vi "Off Mode Standby Mode Power Measure SM.vi"(0 "Equipment":T3, 1 "CDAQ Tasks":refnum<k21>[](array[refnum]), 11 "Error In":errorcluster) -> (4 "Off Mode Watts":dbl, 6 "2015 Output":bool, 8 "Standby Watts":dbl, 10 "Low Power Switch":bool=TRUE, 15 "Error Out":errorcluster)   [LabVIEW 2013]
uses:
  Type Definitions/Equipment DPT.ctl
  Type Definitions/WT500 Sequences.ctl
  <vilib>/Analysis/NI_AALBase.lvlib
panel:
  in  "Main Tab":enum32{"Collecting", "Analyzed"}(tab)
  in  "stop":bool
  out "Power Chart":dbl(graph)
  out "Power (Watts)":dbl
  in  "Skip Standby":bool
  in  "2015 DOE":bool
  out "Off Mode Watts":T1(graph)
  out "5% of Max.":dbl
  out "Max Value.":dbl
  out "Standard Deviation.":dbl
  out "Standby Mode Watts":T1(graph)
  out "Standard Deviation":dbl
  out "Max Value":dbl
  out "5% of Max":dbl
  in  "Complete Test":bool
  in  "Restart":bool
  out "Stable?":bool
  out "Time Sum 4":dbl
  out "Time Sum 3":dbl
  out "Time Sum 2":dbl
  out "Time Sum 1":dbl
  in  "Tab Control":enum32{"Input Parameters", "Debug", "Raw Data"}(tab)
  in  "Processed Data":bool
  in  "Tab Control 2":T2(tab)
  in  "10 Min Power":dbl=600.0
  in  "35 Min":dbl=2100.0
  in  "5 Min Timer":dbl=300.0
  in  "2015?":bool
  out "Current State":string
  in  "High State Timer":dbl=10.0
  out "High Power":dbl
  in  "Low State Timer (5 min)":dbl=300.0
  out "Power Threshold":dbl
  in  "Testing":bool
  in  "Test Power":dbl
  in  "Debug?":bool=TRUE
  out "Debug State":string[](array[string])
  out "DOE Data":dbl[][](array[numeric])
  out "35 Min Data":dbl[][](array[numeric])
  out "Power Threshold Array":dbl[][](array[numeric])
  out "Timer":dbl format="%<%H:%M:%S>t"
  out "String":string
  # "Measure off mode and standby mode for DOE 2015. Reference ETP 112D026 - 2015 DOE Dryer Energy"
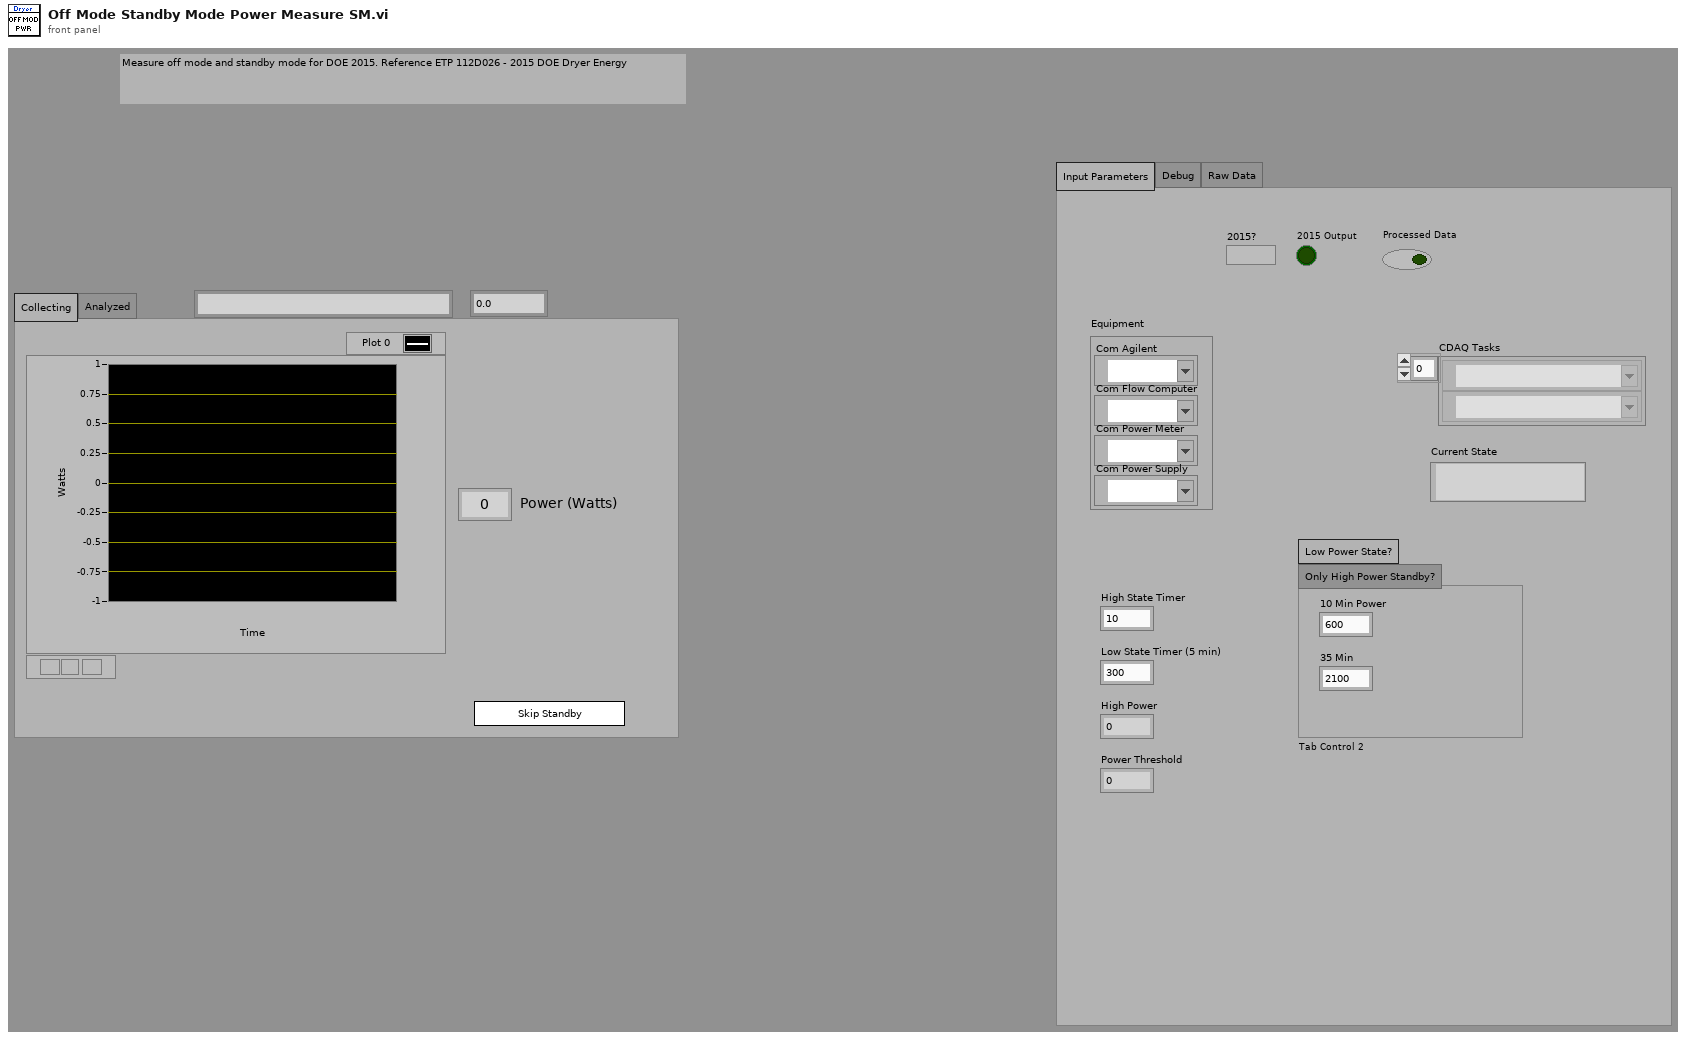
[diagram p1: front panel]
types:
  T1 = cluster{"X Values":dbl[], "Histogram: h(x)":i32[]}
  T2 = enum32{"Low Power State?", "Only High Power Standby?"}
  T3 = typedef "Equipment DPT.ctl" = cluster{"Com Agilent":refnum<visa-resource-name>, "Com Flow Computer":refnum<visa-resource-name>, "Com Power Meter":refnum<visa-resource-name>, "Com Power Supply":refnum<visa-resource-name>}
  T4 = enum32{"invalid app kind", "Development System", "Run Time System", "Student Edition", "Embedded LabVIEW", "Evaluation", "Custom"}
  T5 = enum16{"Exe", "Init CDAQ", "Gather DATA", "Close"}
  T6 = enum32{"Invalid", "Standard", "Closed", "Hidden", "Minimized", "Maximized"}
  T7 = typedef "WT500 Sequences.ctl" = enum16{"Initialize", "GetReadings", "GetErrors", "Close", "NoOp", "MiscCmd"}
  T8 = cluster{"Core":cluster{"Current VI Reference":refnum<vi>, "Close Panel on Exit?":bool}, "Agilent Channel List":string, "Equipment":T3, "T0":dbl, "Tstart":dbl, "Temps":dbl[], "2015?":bool, "CDAQ Tasks":refnum<k21>[], "Labels":string[], "35 Min Data Array":dbl[], "10 Min Data Array":dbl[], "Low Power State?":bool, "Output Data":cluster{"Standard Deviation":dbl, "Off Mode Watts":dbl, "Max Value":dbl, "5% of Max":dbl, "Standby Watts":dbl, "Standard Deviation.":dbl, "Max Value.":dbl, "5% of Max.":dbl}, "Power Threshold":dbl[], "Processed Data":bool, "Main Tab":enum32{"Collecting", "Analyzed"}}
  T9 = cluster{"Standard Deviation":dbl, "Off Mode Watts":dbl, "Max Value":dbl, "5% of Max":dbl, "Standby Watts":dbl, "Standard Deviation.":dbl, "Max Value.":dbl, "5% of Max.":dbl}
  T10 = cluster{"Current VI Reference":refnum<vi>, "Close Panel on Exit?":bool}
  T11 = typedef "Dryer PowerData.ctl" = cluster{"Current L1":dbl, "Current L2":dbl, "Power":dbl, "WattHours":dbl}
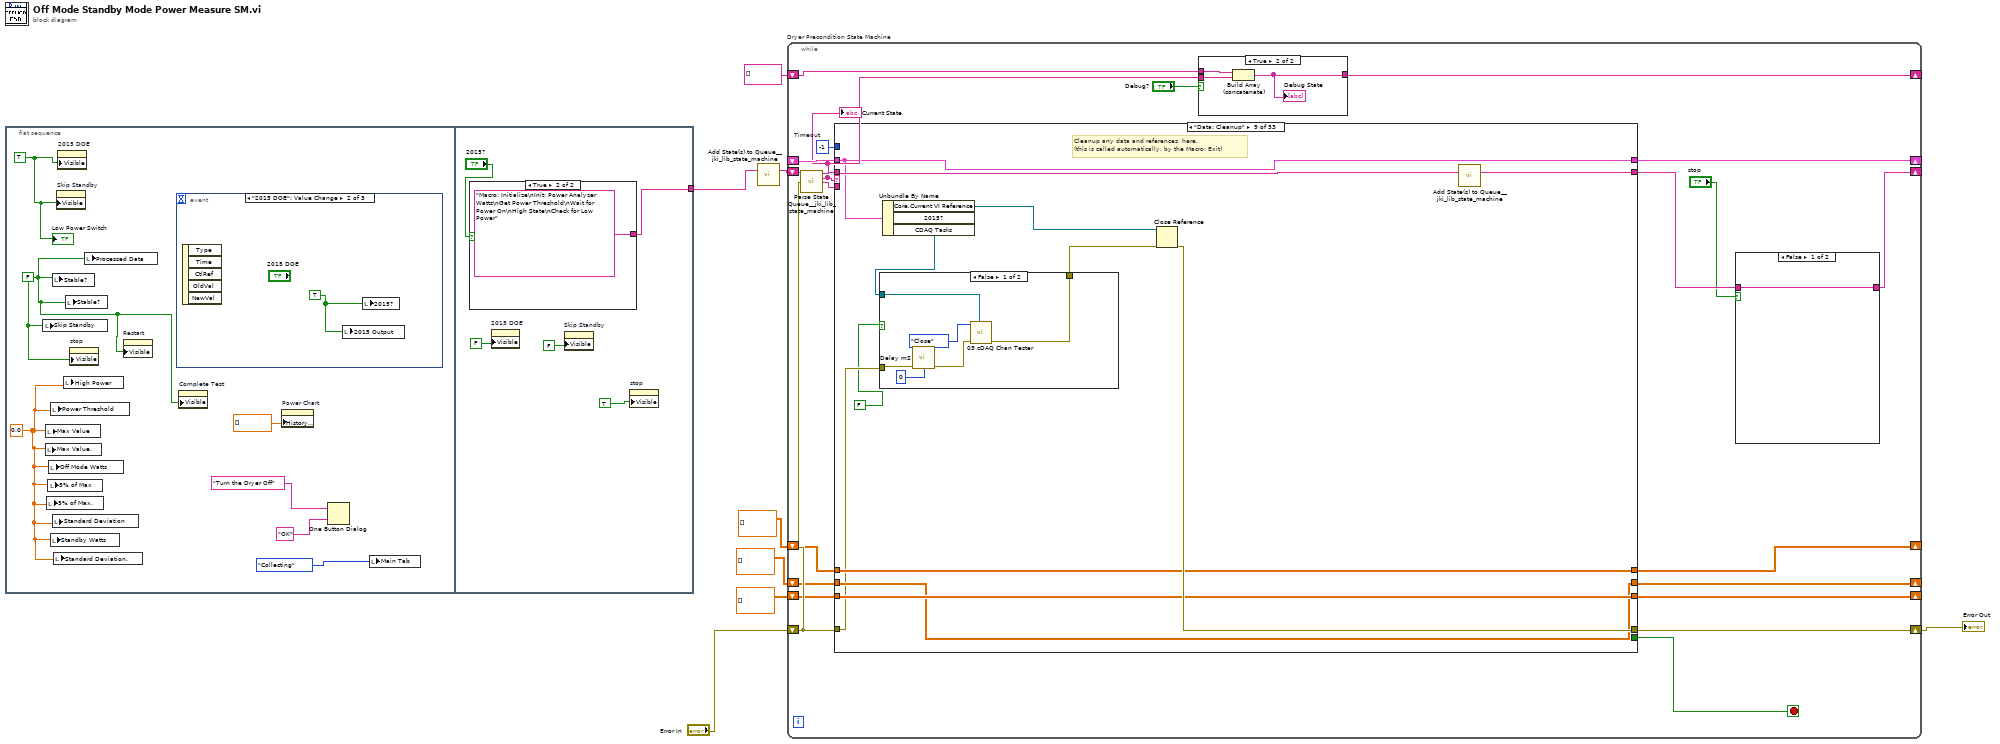
[diagram p0: block diagram]
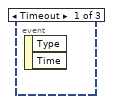
[diagram p2: hidden frame]
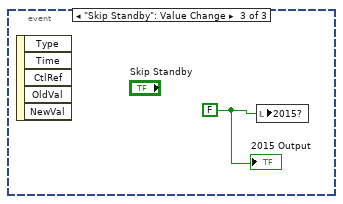
[diagram p3: hidden frame]
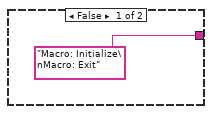
[diagram p4: hidden frame]
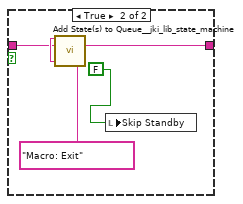
[diagram p5: hidden frame]
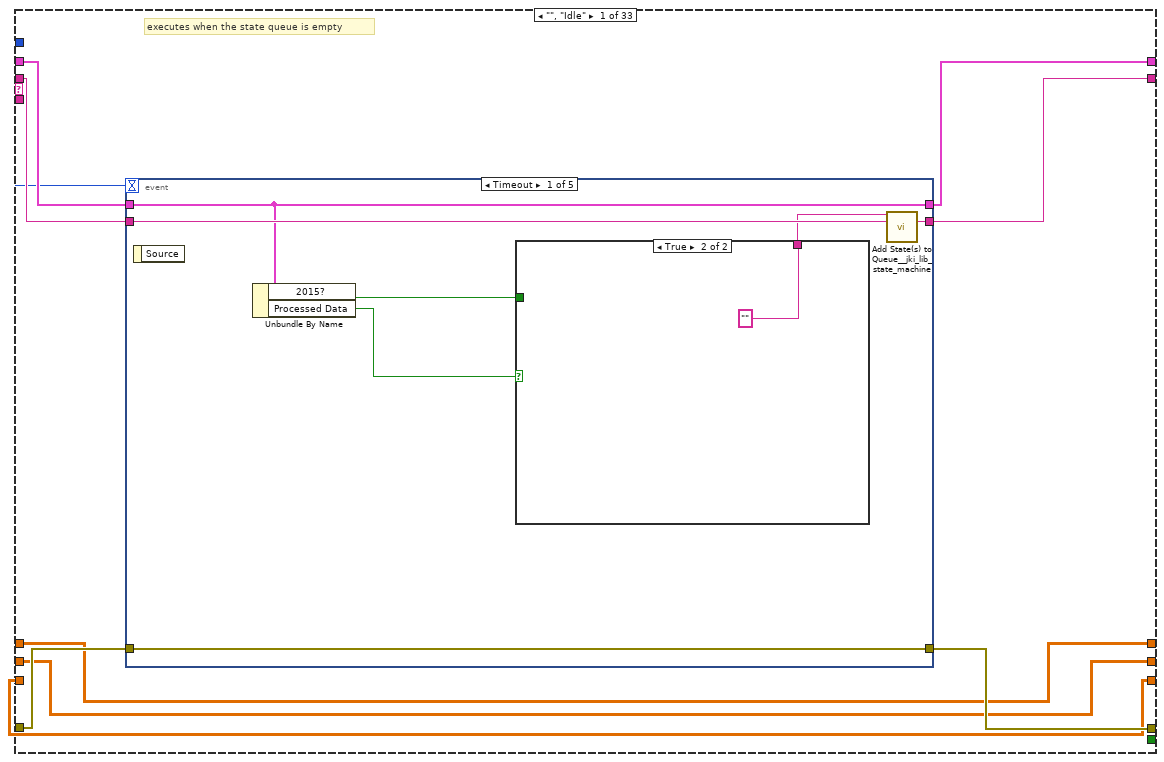
[diagram p7: hidden frame]
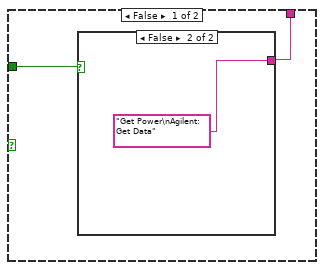
[diagram p8: hidden frame]
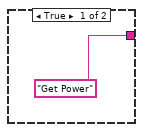
[diagram p9: hidden frame]
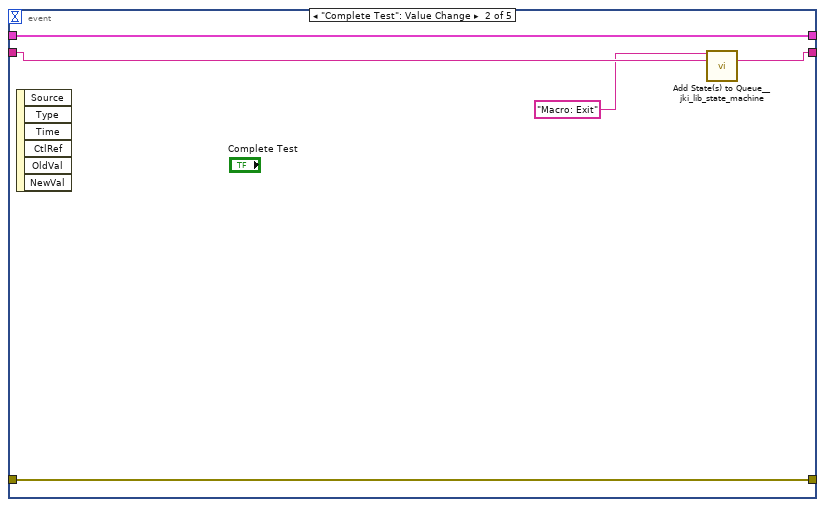
[diagram p10: hidden frame]
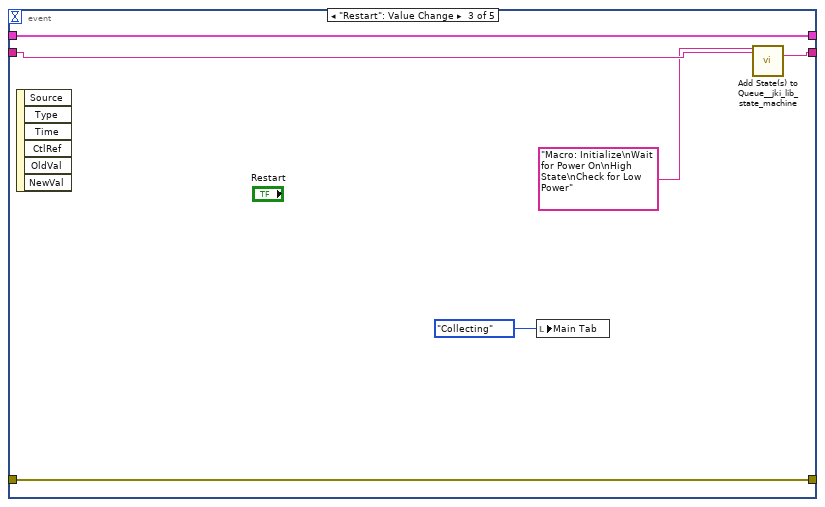
[diagram p11: hidden frame]
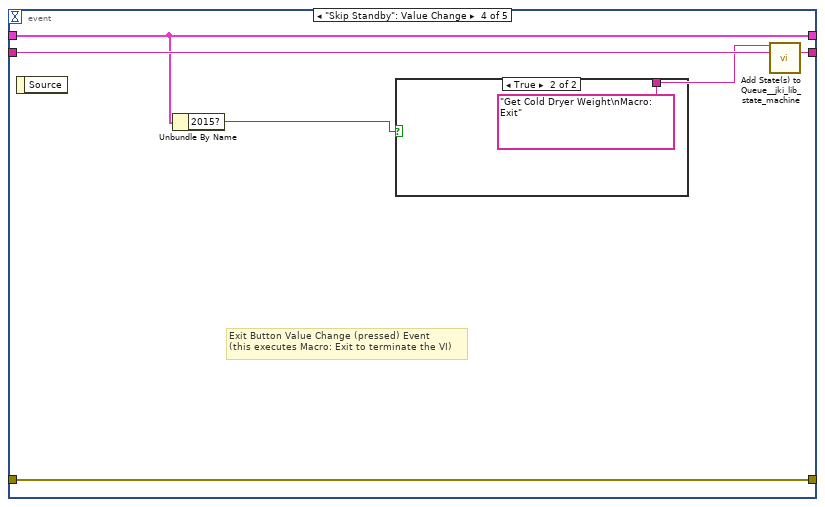
[diagram p12: hidden frame]
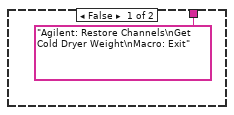
[diagram p13: hidden frame]
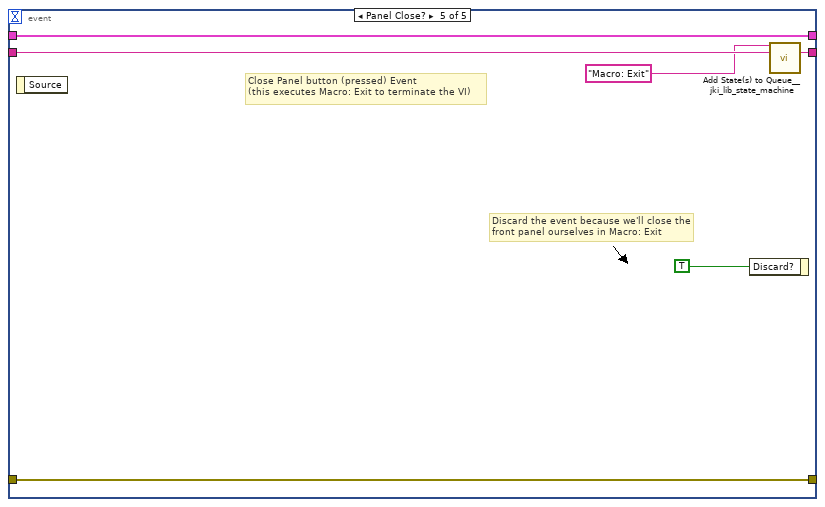
[diagram p14: hidden frame]
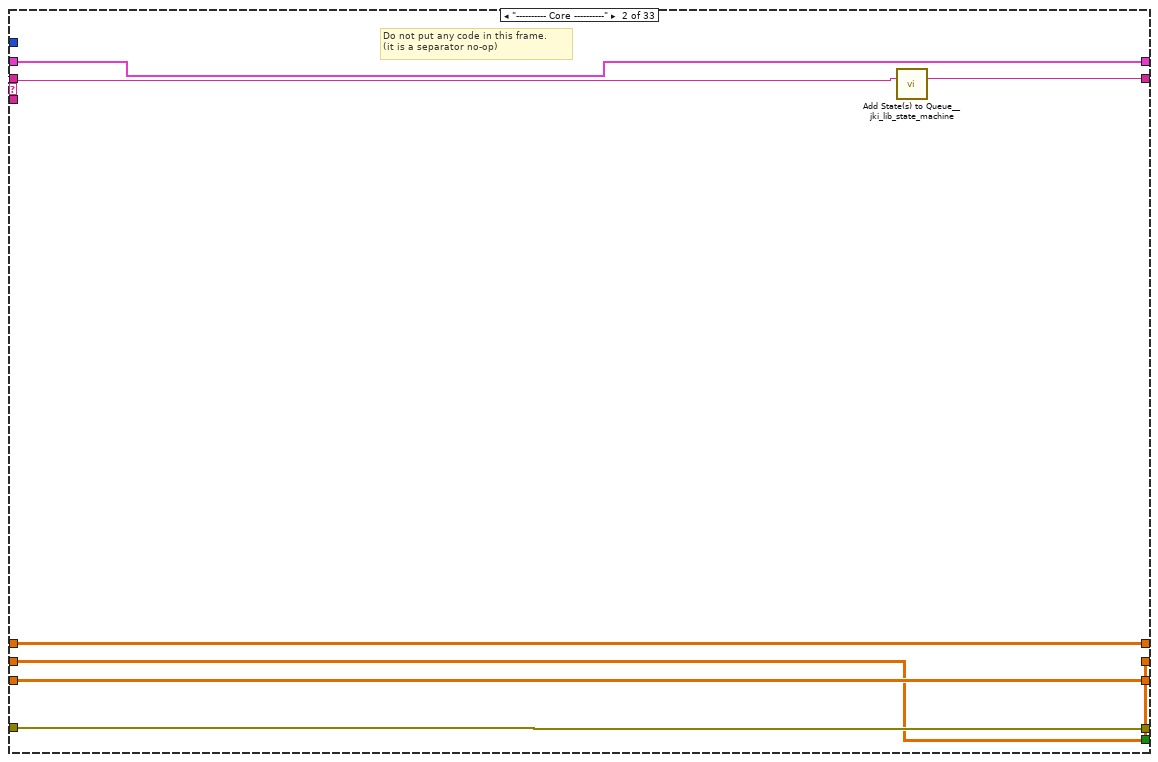
[diagram p15: hidden frame]
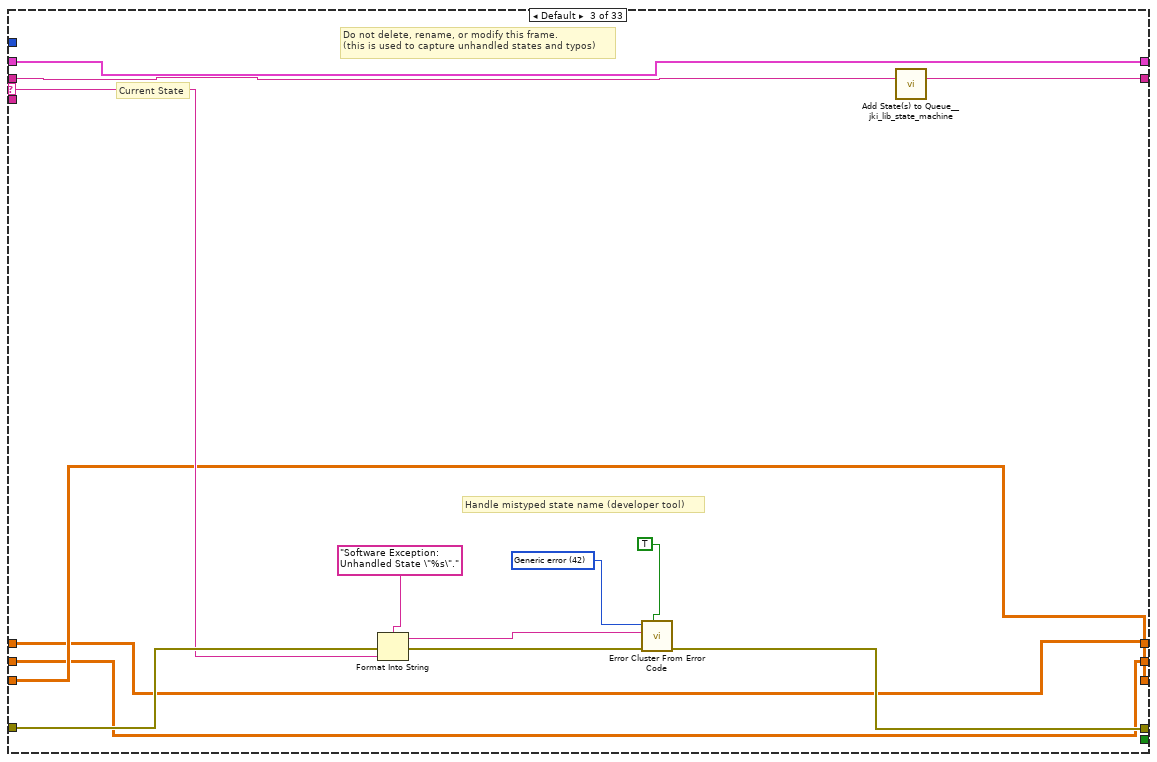
[diagram p16: hidden frame]
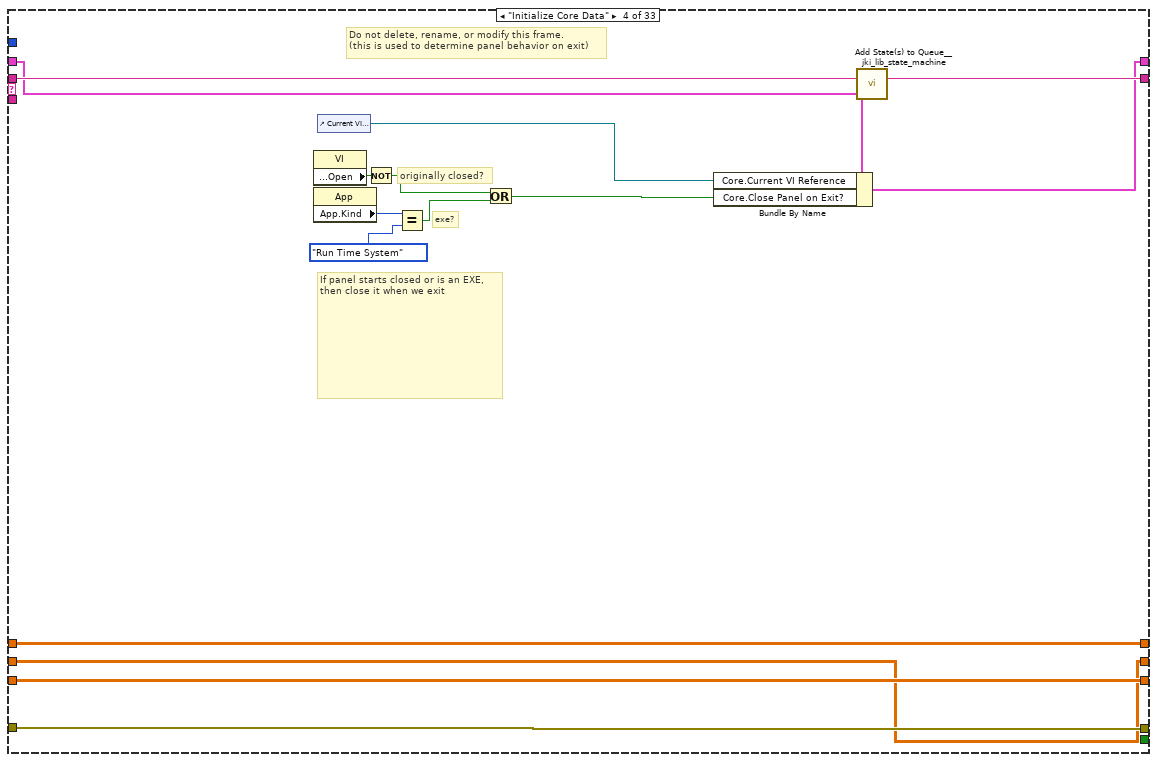
[diagram p17: hidden frame]
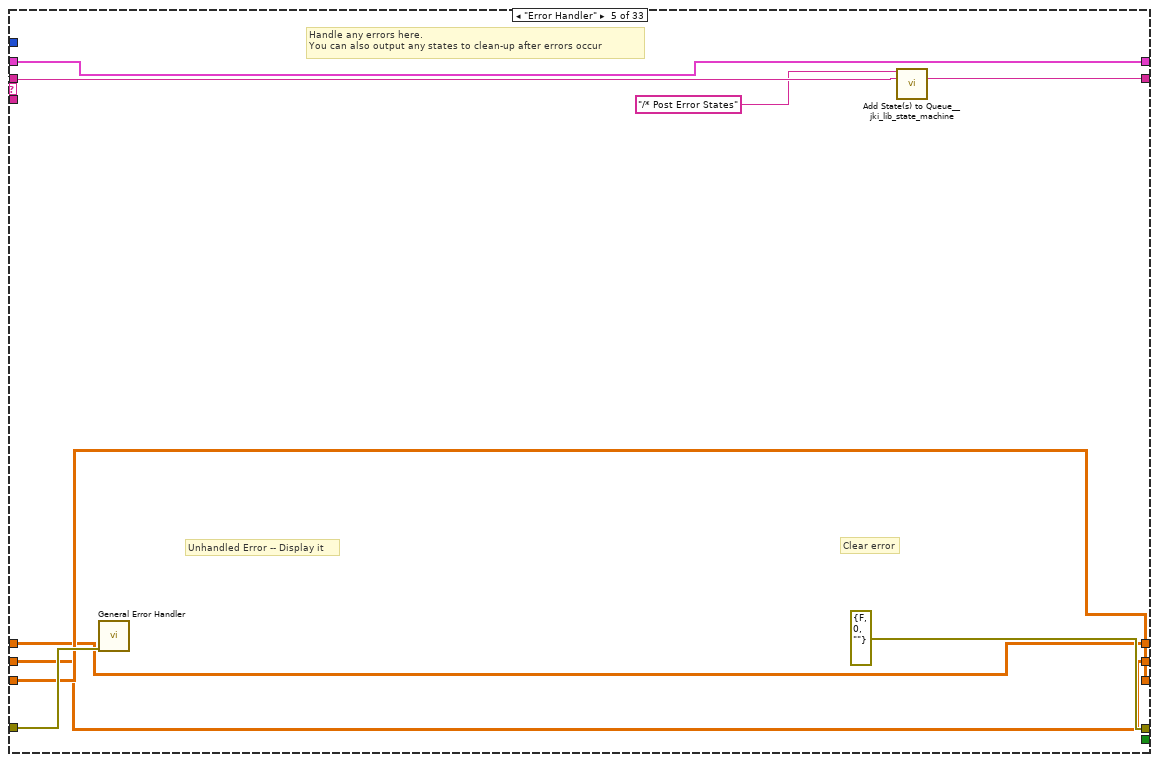
[diagram p18: hidden frame]
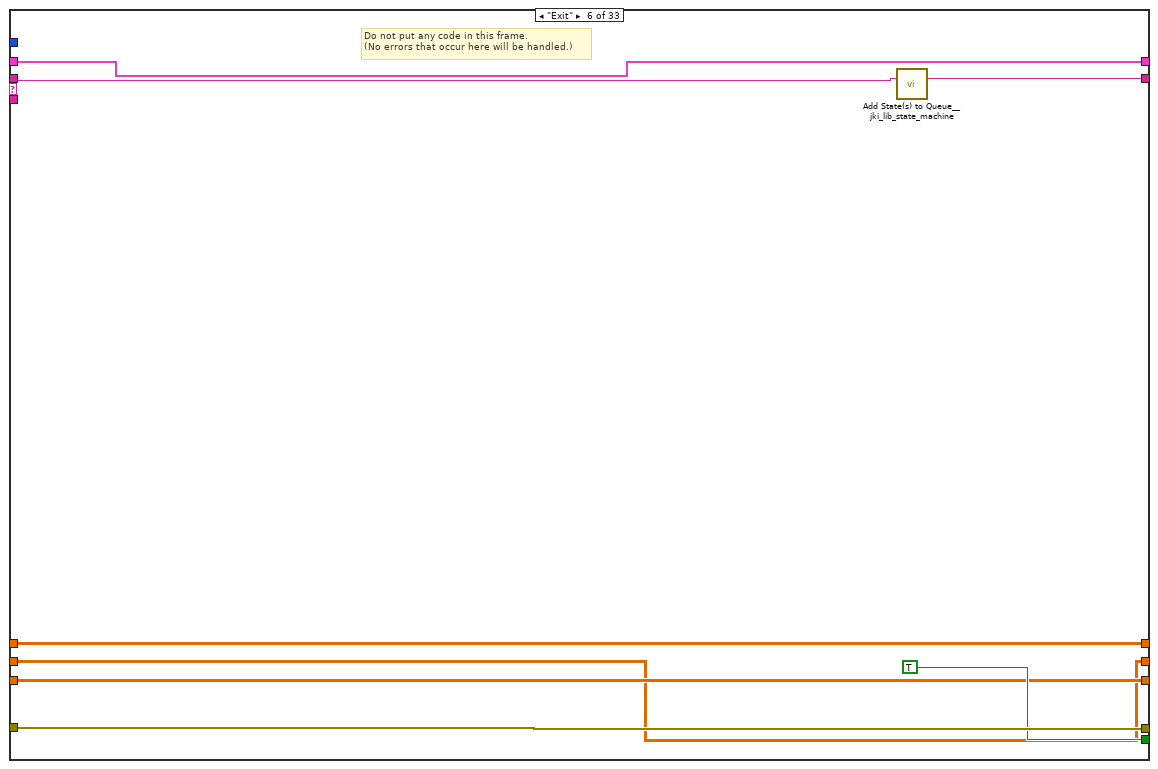
[diagram p19: hidden frame]
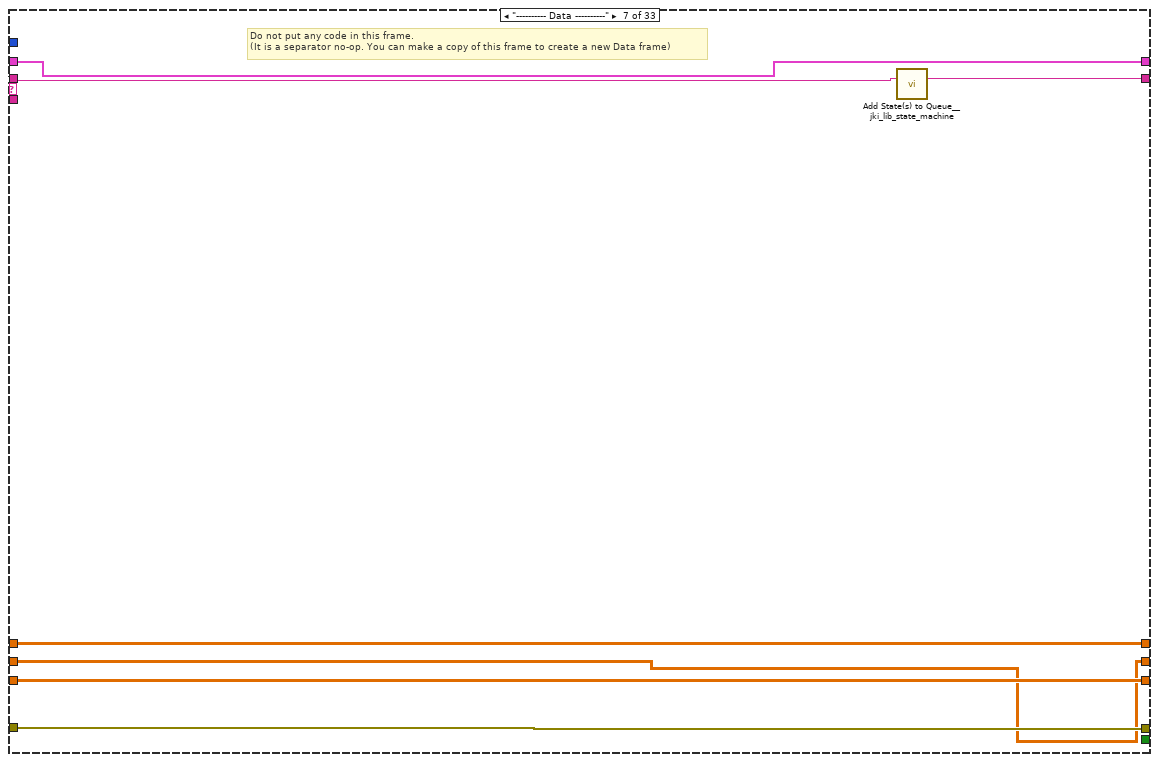
[diagram p20: hidden frame]
diagram:
  n1 = flat-sequence {
    tunnel: [w22] -> w7
    frame #0 {
      w12 = 0.0 ("Max Value")
      w10 = FALSE ("Off Mode Stable?")
      w11 = TRUE ("Visible")
      n2 = local write "Skip Standby"(w10) -> ()
      n3 = local write "Max Value."(w12) -> ()
      n4 = local write "Max Value"(w12) -> ()
      n5 = local write "5% of Max."(w12) -> ()
      n6 = local write "5% of Max"(w12) -> ()
      n7 = local write "Off Mode Watts"(w12) -> ()
      n8 = local write "Standby Watts"(w12) -> ()
      n9 = local write "Power Threshold"(w12) -> ()
      n10 = local write "Stable?"(w10) -> ()
      n11 = local write "Standard Deviation"(w12) -> ()
      n12 = local write "Standard Deviation."(w12) -> ()
      n13 = property on="Skip Standby" class="Bool (strict)"("Visible"=w11) -> ()  [unwired: 2 in, 2 out]
      n14 = property on="2015 DOE" class="Bool (strict)"("Visible"=w11) -> ()  [unwired: 2 in, 2 out]
      n15 = local write "High Power"(w12) -> ()
      n16 = local write "Stable?"(w10) -> ()
      n17 = property on="stop" class="Bool (strict)"("Visible"=w10) -> ()  [unwired: 2 in, 2 out]
      n18 = local write "Processed Data"(w10) -> ()
      n19 = property on="Restart" class="Bool (strict)"("Visible"=w10) -> ()  [unwired: 2 in, 2 out]
      n20 = event shown="[1] \"2015 DOE\": Value Change" {
        selector: _ -> [_ _ _]
        dyn-events: _ -> [_ _ _]
        timeout: _ -> [_ _ _]
        event Timeout {
          n21 = event-data() -> ()  [unwired: 1 in, 2 out]
        }
        event "2015 DOE": Value Change {
          w16 = TRUE ("CDAQ?")
          n22 = event-data() -> ()  [unwired: 1 in, 5 out]
          n23 = local write "2015 Output"(w16) -> ()
          n24 = local write "2015?"(w16) -> ()
        }
        event "Skip Standby": Value Change {
          w17 = FALSE ("2015?")
          n25 = event-data() -> ()  [unwired: 1 in, 5 out]
          n26 = local write "2015?"(w17) -> ()
          "2015 Output" <- w17
        }
      }
      n27 = property on="Complete Test" class="Bool (strict)"("Visible"=w10) -> ()  [unwired: 2 in, 2 out]
      n28 = property on="Power Chart" class="WFChart (strict)"("History Data"=dbl[] []) -> ()  [unwired: 2 in, 2 out]
      n29 = One Button Dialog(message="Turn the Dryer Off", button name ("OK")="OK") -> ()  [unwired: 1 out]
      n30 = local write "Main Tab"(enum32{"Collecting", "Analyzed"}."Collecting" ("Tab Control 3")) -> ()
      "Low Power Switch" <- w11
    }
    frame #1 {
      n31 = case shown="True" "2015?" {
        tunnel: ["Macro: Initialize\nMacro: Exit" "Macro: Initialize\nInit: Power Analyzer Watts\nGet Power Threshold\nWait for Power On\nHigh State\nCheck for Low Power"] -> w22
        frame False {
        }
        frame True {
        }
      }
      n32 = property on="2015 DOE" class="Bool (strict)"("Visible"=FALSE) -> ()  [unwired: 2 in, 2 out]
      n33 = property on="Skip Standby" class="Bool (strict)"("Visible"=FALSE) -> ()  [unwired: 2 in, 2 out]
      n34 = property on="stop" class="Bool (strict)"("Visible"=TRUE) -> ()  [unwired: 2 in, 2 out]
    }
  }
  n35 = call <vilib>:"Add State(s) to Queue__jki_lib_state_machine.vi"("State(s) in (\"\")"=w7) -> ("States Out"=w8:string)  [unwired: 14 in]
  n36 = while "Dryer Precondition State Machine" {
    shift-right: [w41] -> _
    shift-left: _ -> [w40]
    shift-right: [w43] -> w5
    shift-left: "Error In" -> [w38]
    shift-right: [w28] -> _
    shift-left: w8 -> [w44]
    shift-right: [w35] -> _
    shift-left: string[] [] -> [w34]
    shift-right: [w32] -> _
    shift-left: dbl[][] [] -> [w33]
    shift-right: [w30] -> _
    shift-left: dbl[][] [] -> [w31]
    shift-right: [w26] -> _
    shift-left: dbl[][] [] -> [w27]
    stop <- w42 stop-if-true
    w39 = -1  # Timeout
    n37 = call <vilib>:"Parse State Queue__jki_lib_state_machine.vi"("State Queue"=w44, "Error In (no error)"=w38) -> ("Remaining States"=w46:string, "Current State"=w36:string, "Arguments"=w45:string)  [unwired: 11 in]
    "Current State" <- w36
    n38 = case shown="\"Data: Cleanup\"" w36 {
      selector: w36 -> [_ _ w113 _ _ _ _ _ _ _ _ _ _ _ _ _ _ w307 w333 _ _ _ _ _ _ _ _ _ _ _ _ _ _]
      tunnel: w46 -> [w65 w109 w117 w138 w147 w155 w162 w187 w199 w213 w220 w229 w243 w272 w280 w293 w300 w314 w340 w359 w376 w418 w452 w489 w536 w576 w613 w650 w687 w737 w781 w799 w819]
      tunnel: w45 -> [_ _ _ _ _ _ _ _ _ _ _ w224 w237 _ _ _ _ _ _ _ _ _ _ _ _ _ _ _ _ _ _ _ _]
      tunnel: w40 -> [w63 w106 w115 w129 w144 w153 w159 _ w195 w210 w218 w227 w239 w269 w277 w290 w297 w310 w336 w356 w373 w415 w449 w486 w533 w573 w610 w647 w684 w706 w776 w797 w814]
      tunnel: [w62 w107 w119 w135 errorcluster {"status"=FALSE, "code"=0, "source"=""} ("error out") w152 w160 w185 w196 w211 w217 w225 w240 w270 w278 w291 w298 w302 w328 w357 w374 w404 w450 w487 w534 w574 w611 w648 w685 w735 w777 w790 w815] -> w43
      tunnel: w38 -> [w61 w107 w118 w135 w143 w152 w160 w185 w191 w211 w217 w226 w241 w270 w278 w291 w298 w308 w334 w357 w374 w404 w450 w487 w534 w574 w611 w648 w685 w735 w775 w791 w815]
      tunnel: [w64 w108 w116 w137 w146 w154 w161 w186 w198 w212 w219 w228 w242 w271 w279 w292 w299 w313 w339 w358 w375 w417 w451 w488 w535 w575 w612 w649 w686 w736 w780 w798 w818] -> w29
      tunnel: [_ _ _ _ _ TRUE _ _ _ _ _ _ _ _ _ _ _ _ _ _ _ _ _ _ _ _ _ _ _ _ _ _ _] -> w42
      tunnel: [w60 w106 w115 w136 w144 w153 w159 w181 w195 w210 w218 w227 w239 w269 w277 w290 w297 w310 w336 w356 w372 w414 w448 w485 w532 w572 w609 w646 w683 w706 w779 w796 w813] -> w41
      tunnel: w39 -> [w59 _ _ _ _ _ _ _ _ _ _ _ _ _ _ _ _ _ _ _ _ _ _ _ _ _ _ _ _ _ _ _ _]
      tunnel: w33 -> [w58 w105 w112 w126 w141 w150 w158 w174 w194 w209 w216 w223 w236 w268 w275 w283 w296 w312 w338 w355 w362 w408 w438 w472 w522 w563 w601 w638 w669 w733 w774 w789 w810]
      tunnel: [w58 w105 w112 w126 w141 w150 w158 w174 w194 w209 w216 w223 w236 w268 w275 w283 w296 w312 w338 w355 w362 w408 w438 w472 w522 w563 w596 w636 w669 w733 w774 w789 w810] -> w32
      tunnel: w31 -> [w57 w104 w111 w125 w140 w149 w157 w171 w193 w208 w215 w222 w235 w267 w274 w282 w295 w311 w337 w354 w364 w407 w440 w477 w518 w561 w599 w635 w674 w732 w773 w788 w809]
      tunnel: [w57 w104 w111 w125 w140 w149 w157 w171 w193 w208 w215 w222 w235 w267 w274 w282 w295 w311 w337 w354 w364 w407 w440 w477 w521 w561 w599 w635 w673 w732 w773 w788 w809] -> w30
      tunnel: w27 -> [w56 w103 w110 w124 w139 w148 w156 w166 w192 w207 w214 w221 w234 w266 w273 w281 w294 w305 w331 w353 w361 w406 w437 w471 w517 w559 w594 w631 w668 w711 w772 w785 w808]
      tunnel: [w56 w103 w110 w124 w139 w148 w156 w166 w192 w207 w214 w221 w234 w266 w273 w281 w294 w305 w331 w353 w360 w406 w437 w471 w517 w559 w594 w631 w668 w711 w772 w785 w808] -> w26
      frame "", "Idle" {
        # "executes when the state queue is empty"
        n39 = event shown="[0] Timeout" {
          selector: _ -> [_ _ _ _ _]
          dyn-events: _ -> [_ _ _ _ _]
          timeout: w59 -> [_ _ _ _ _]
          tunnel: w65 -> [w72 w81 w86 w94 w102]
          tunnel: [w71 w79 w87 w93 w101] -> w64
          tunnel: w63 -> [w68 w82 w88 w90 w99]
          tunnel: [w70 w78 w84 w92 w100] -> w62
          tunnel: w61 -> [w70 w78 w84 w92 w100]
          tunnel: [w68 w82 w88 w90 w99] -> w60
          event Timeout {
            n40 = event-data() -> ()  [unwired: 1 in, 1 out]
            n41 = Unbundle By Name(w68) -> ("2015?"=w67:bool, "Processed Data"=w66:bool)
            n42 = case shown="True" w66 {
              tunnel: [w74 "" ("State(s) in Front (\"\")")] -> w69
              tunnel: w67 -> [w73 _]
              frame False {
                n43 = case shown="False" w73 {
                  tunnel: ["Get Power" ("State(s) in Front (\"\")") "Get Power\nAgilent: Get Data" ("State(s) in Front (\"\")")] -> w74
                  frame True {
                  }
                  frame False {
                  }
                }
              }
              frame True {
              }
            }
            n44 = call <vilib>:"Add State(s) to Queue__jki_lib_state_machine.vi"("State(s) in Front (\"\")"=w69, "State(s) in (\"\")"=w72) -> ("States Out"=w71:string)  [unwired: 13 in]
          }
          event "Complete Test": Value Change {
            n45 = event-data() -> ()  [unwired: 1 in, 6 out]
            n46 = call <vilib>:"Add State(s) to Queue__jki_lib_state_machine.vi"("State(s) in Front (\"\")"="Macro: Exit", "State(s) in (\"\")"=w81) -> ("States Out"=w79:string)  [unwired: 13 in]
          }
          event "Restart": Value Change {
            n47 = event-data() -> ()  [unwired: 1 in, 6 out]
            n48 = local write "Main Tab"(enum32{"Collecting", "Analyzed"}."Collecting" ("Main Tab")) -> ()
            n49 = call <vilib>:"Add State(s) to Queue__jki_lib_state_machine.vi"("State(s) in Front (\"\")"="Macro: Initialize\nWait for Power On\nHigh State\nCheck for Low Power", "State(s) in (\"\")"=w86) -> ("States Out"=w87:string)  [unwired: 13 in]
          }
          event "Skip Standby": Value Change {
            # "Exit Button Value Change (pressed) Event\n(this executes Macro: Exit to terminate the VI)"
            n50 = event-data() -> ()  [unwired: 1 in, 1 out]
            n51 = Unbundle By Name(w90) -> ("2015?"=w89:bool)
            n52 = case shown="True" w89 {
              tunnel: ["Agilent: Restore Channels\nGet Cold Dryer Weight\nMacro: Exit" "Get Cold Dryer Weight\nMacro: Exit"] -> w91
              frame False {
              }
              frame True {
              }
            }
            n53 = call <vilib>:"Add State(s) to Queue__jki_lib_state_machine.vi"("State(s) in Front (\"\")"=w91, "State(s) in (\"\")"=w94) -> ("States Out"=w93:string)  [unwired: 13 in]
          }
          event Panel Close? {
            # "Discard the event because we'll close the front panel ourselves in Macro: Exit"
            # "Close Panel button (pressed) Event\n(this executes Macro: Exit to terminate the VI)"
            n54 = event-data() -> ()  [unwired: 1 in, 1 out]
            n55 = event-data("Discard?"=TRUE) -> ()  [unwired: 1 in, 1 out]
            n56 = call <vilib>:"Add State(s) to Queue__jki_lib_state_machine.vi"("State(s) in Front (\"\")"="Macro: Exit", "State(s) in (\"\")"=w102) -> ("States Out"=w101:string)  [unwired: 13 in]
          }
        }
      }
      frame "---------- Core ----------" {
        # "Do not put any code in this frame.\n(it is a separator no-op)"
        n57 = call <vilib>:"Add State(s) to Queue__jki_lib_state_machine.vi"("State(s) in (\"\")"=w109) -> ("States Out"=w108:string)  [unwired: 14 in]
      }
      frame Default {
        w122 = 42 items=["No error", "Argument error", "Memory is full", "Out of zone", "End of file", "File already open", "Generic file I/O error", "File not found", "File permission error", "Disk is full", "Duplicate path", "Too many files open", "System feature not enabled", "Resource file not found", "Cannot add resource", "Resource not found", "Image not found", "Image memory error", "Pen does not exist", "Config type invalid", "Config token not found", "Config parse error", "Config memory error", "Bad external code format", "Bad external code offset", "External code not present", "Null window", "Destroy window error", "Null menu", "Print aborted", "Bad print record", "Print driver error", "Windows error during printing", "Memory error during printing", "Print dialog error", "Generic print error", "Invalid device refnum", "Device not found", "Device parameter error", "Device unit error", "Cannot open device", "Device call aborted", "Generic error", "Cancelled by user", "Object ID too low", "Object ID too high", "Object not in heap", "Unknown heap", "Unknown object (invalid DefProc)", "Unknown object (DefProc not in table)", "Message out of range", "Invalid (null) method", "Unknown message", "Manager call not supported", "Bad address", "Network operation in progress", "Network operation timed out", "Connection is busy", "Network attribute not supported", "Network error", "Address in use", "System out of memory", "Connection aborted", "Connection refused", "Not connected", "Already connected", "Connection closed", "Initialization error (interapplication manager)", "Bad occurrence", "Wait on unbound occurrence handler", "Occurrence queue overflow", "Datalog type conflict", "Unused", "Unrecognized type (interapplication manager)", "Memory corrupt", "Failed to make temporary DLL", "Old CIN version", "Drag socket not found", "Failed to load drop-object", "Failed to register OLE object", "Failed to release OLE object", "Format specifier type mismatch", "Unknown format specifier", "Too few format specifiers", "Too many format specifiers", "Scan failed", "Newer CIN version", "Error converting to variant", "Runtime menu error", "Password tampered", "Variant attribute not found", "Incompatible variant data type", "Event data is not available", "Event Store is not present", "Occurrence is not found", "Event Queue is not created", "Event info is not available", "Refnum passed is NULL", "Error retrieving Class GUID", "Error retrieving CoClass GUID", "Error retrieving TypeLib GUID.", "Bad built application magic bytes.", "Specific driver is different from the specific driver associated with the Logical Name.", "There is no session opened to the class driver.", "Max Error", "MAX - Error with config objects", "MAX - Error loading configuration", "MAX - Group not supported"]
        # "Current State"
        # "Do not delete, rename, or modify this frame.\n(this is used to capture unhandled states and typos)"
        # "Handle mistyped state name (developer tool)"
        n58 = Format Into String(format string="Software Exception: Unhandled State \"%s\"." ("message"), error in=w118, w113) -> (resulting string=w121:string, error out=w120:errorcluster)  [unwired: 1 in]
        n59 = call <vilib>:"Error Cluster From Error Code.vi"("show call chain? (False)"=TRUE, "error in (no error)"=w120, "error message (\"\")"=w121, "error code (0)"=w122) -> ("error out"=w119:errorcluster)  [unwired: 5 in]
        n60 = call <vilib>:"Add State(s) to Queue__jki_lib_state_machine.vi"("State(s) in (\"\")"=w117) -> ("States Out"=w116:string)  [unwired: 14 in]
      }
      frame "Initialize Core Data" {
        # "Do not delete, rename, or modify this frame.\n(this is used to determine panel behavior on exit)"
        # "originally closed?"
        # "exe?"
        # "If panel starts closed or is an EXE, then close it when we exit"
        n61 = property class="VI"() -> ("Front Panel.Open"=w134:bool)  [unwired: 2 in, 2 out]
        n62 = property class="App"() -> ("App.Kind"=w133:T4)  [unwired: 2 in, 2 out]
        n63 = control-ref of="Current VI Reference"() -> (w127:refnum<vi>)
        n64 = Not(x=w134) -> (.not. x?=w131:bool)
        n65 = Equal?(x=w133, y=T4."Run Time System" ("Application:Kind")) -> (x = y?=w130:bool)
        n66 = Or(x=w131, y=w130) -> (x .or. y?=w128:bool)
        n67 = Bundle By Name(cluster=w129, "Core.Current VI Reference"=w127, "Core.Close Panel on Exit?"=w128) -> (w136:T8)
        n68 = call <vilib>:"Add State(s) to Queue__jki_lib_state_machine.vi"("State(s) in (\"\")"=w138) -> ("States Out"=w137:string)  [unwired: 14 in]
      }
      frame "Error Handler" {
        # "Unhandled Error -- Display it"
        # "Handle any errors here.\nYou can also output any states to clean-up after errors occur"
        # "Clear error"
        n69 = call <vilib>:"General Error Handler.vi"("error in (no error)"=w143) -> ()  [unwired: 10 in, 5 out]
        n70 = call <vilib>:"Add State(s) to Queue__jki_lib_state_machine.vi"("State(s) in Front (\"\")"="/* Post Error States", "State(s) in (\"\")"=w147) -> ("States Out"=w146:string)  [unwired: 13 in]
      }
      frame "Exit" {
        # "Do not put any code in this frame.\n(No errors that occur here will be handled.)"
        n71 = call <vilib>:"Add State(s) to Queue__jki_lib_state_machine.vi"("State(s) in (\"\")"=w155) -> ("States Out"=w154:string)  [unwired: 14 in]
      }
      frame "---------- Data ----------" {
        # "Do not put any code in this frame.\n(It is a separator no-op. You can make a copy of this frame to create a new Data frame)"
        n72 = call <vilib>:"Add State(s) to Queue__jki_lib_state_machine.vi"("State(s) in (\"\")"=w162) -> ("States Out"=w161:string)  [unwired: 14 in]
      }
      frame "Data: Initialize" {
        w167 = dbl[] []  # Power Threshold
        w168 = T9 {"Standard Deviation"=0.0, "Off Mode Watts"=0.0, "Max Value"=0.0, "5% of Max"=0.0, "Standby Watts"=0.0, "Standard Deviation."=0.0, "Max Value."=0.0, "5% of Max."=0.0}  # Output Data
        w169 = FALSE  # Low Power State?
        w170 = 0.0 ("Timer")
        w172 = dbl[] []  # 10 Min Data Array
        w173 = dbl[] []  # 35 Min Data Array
        w175 = string[] []  # Labels
        w178 = dbl[] []  # Temps
        w179 = 0.0  # Tstart
        w180 = 0.0  # T0
        w182 = ""  # Agilent Channel List
        w184 = T10 {"Current VI Reference"=refnum, "Close Panel on Exit?"=TRUE}  # Core
        # "Initialize the shift-register data, here.\n(data names are defined by what you wire into the bundle function)"
        n73 = local read "2015?"() -> (w177:bool)
        n74 = local write "Power (Watts)"(w170) -> ()
        n75 = local write "Timer"(w170) -> ()
        n76 = local write "Processed Data"(FALSE ("Processed Data")) -> ()
        n77 = Bundle("Core"=w184, "Agilent Channel List"=w182, "Equipment"="Equipment", "T0"=w180, "Tstart"=w179, "Temps"=w178, "2015?"=w177, "CDAQ Tasks"="CDAQ Tasks", "Labels"=w175, "35 Min Data Array"=w173, "10 Min Data Array"=w172, "Low Power State?"=w169, "Output Data"=w168, "Power Threshold"=w167, "Processed Data"="Processed Data", "Main Tab"="Main Tab") -> (w181:T8)  [unwired: 1 in]
        n78 = call <vilib>:"Add State(s) to Queue__jki_lib_state_machine.vi"("State(s) in (\"\")"=w187) -> ("States Out"=w186:string)  [unwired: 14 in]
      }
      frame "Data: Cleanup" {
        # "Cleanup any data and references, here.\n(this is called automatically, by the Macro: Exit)"
        n79 = Unbundle By Name(w195) -> ("Core.Current VI Reference"=w197:refnum<vi>, "CDAQ Tasks"=w189:refnum<k21>[])  [unwired: 1 out]
        n80 = case shown="False" FALSE {
          tunnel: w191 -> [w201 w206]
          tunnel: [w205 w206] -> w190
          tunnel: w189 -> [w200 _]
          frame False {
            n81 = call "Delay mS.vi"("Error In"=w201, "milliseconds to wait"=u32 0) -> ("Error Out"=w203:errorcluster)  [unwired: 13 in]
            n82 = call "03 cDAQ Chan Tester.vi"("Tasks In"=w200, "error in (no error)"=w203, "Mode"=T5."Close") -> ("error out"=w205:errorcluster)  [unwired: 6 in, 2 out]
          }
          frame True {
          }
        }
        n83 = Close Reference(reference=w197, error in (no error)=w190) -> (error out=w196:errorcluster)
        n84 = call <vilib>:"Add State(s) to Queue__jki_lib_state_machine.vi"("State(s) in (\"\")"=w199) -> ("States Out"=w198:string)  [unwired: 14 in]
      }
      frame "---------- UI ----------" {
        # "Do not put any code in this frame.\n(It is a separator no-op. You can make a copy of this frame to create a new UI frame)"
        n85 = call <vilib>:"Add State(s) to Queue__jki_lib_state_machine.vi"("State(s) in (\"\")"=w213) -> ("States Out"=w212:string)  [unwired: 14 in]
      }
      frame "UI: Initialize" {
        # "Initialize the User Interface, here.\n(this is called automatically, by the Macro: Init)"
        n86 = call <vilib>:"Add State(s) to Queue__jki_lib_state_machine.vi"("State(s) in (\"\")"=w220) -> ("States Out"=w219:string)  [unwired: 14 in]
      }
      frame "UI: Cursor Set" {
        # "Argument"
        # "Set and Unset Cursor Busy.\n(Usage: \"UI: Cursor Set >> Busy|Idle\")"
        n87 = case shown="\"Idle\", Default" w224 {
          tunnel: w226 -> [w231 w233]
          tunnel: [w230 w232] -> w225
          frame "Idle", Default {
            n88 = call <vilib>:"Unset Busy.vi"("error in (no error)"=w231) -> ("error out"=w230:errorcluster)  [unwired: 10 in]
          }
          frame "Busy" {
            n89 = call <vilib>:"Set Busy.vi"("error in (no error)"=w233) -> ("error out"=w232:errorcluster)  [unwired: 9 in, 1 out]
          }
        }
        n90 = call <vilib>:"Add State(s) to Queue__jki_lib_state_machine.vi"("State(s) in (\"\")"=w229) -> ("States Out"=w228:string)  [unwired: 14 in]
      }
      frame "UI: Front Panel State" {
        # "Argument"
        # "Set Front Panel Open or Closed\n(Usage: \"UI: Front Panel State >> Open|Close\")"
        n91 = Unbundle By Name(w239) -> ("Core.Current VI Reference"=w238:refnum<vi>)
        n92 = case shown="\"Open\", Default" w237 {
          tunnel: w241 -> [w247 w260]
          tunnel: [w249 w261] -> w240
          tunnel: w238 -> [w248 w258]
          frame "Open", Default {
            n93 = property class="VI"(reference=w248, error in=w247) -> (reference out=w245:refnum<vi>, error out=w246:errorcluster, "Front Panel.Open"=w244:bool)
            n94 = case shown="True" w244 {
              tunnel: [w252 w255] -> w249
              tunnel: w246 -> [w251 w255]
              tunnel: w245 -> [w250 _]
              frame False {
                n95 = invoke class="VI" method="FP.Open"(reference=w250, error in=w251, "Activate"=TRUE, "State"=T6."Standard") -> (error out=w252:errorcluster)  [unwired: 1 in, 4 out]
              }
              frame True {
              }
            }
          }
          frame "Close" {
            n96 = property class="VI"(reference=w258, error in=w260) -> (reference out=w257:refnum<vi>, error out=w259:errorcluster, "Front Panel.Open"=w256:bool)
            n97 = case shown="True" w256 {
              tunnel: [w262 w265] -> w261
              tunnel: w259 -> [w262 w264]
              tunnel: w257 -> [_ w263]
              frame False {
              }
              frame True {
                n98 = invoke class="VI" method="FP.Close"(reference=w263, error in=w264) -> (error out=w265:errorcluster)  [unwired: 1 in, 2 out]
              }
            }
          }
        }
        n99 = call <vilib>:"Add State(s) to Queue__jki_lib_state_machine.vi"("State(s) in (\"\")"=w243) -> ("States Out"=w242:string)  [unwired: 14 in]
      }
      frame "---------- Macro ----------" {
        # "Do not put any code in this frame.\n(It is a separator no-op. You can make a copy of this frame to create a new Macro frame)"
        n100 = call <vilib>:"Add State(s) to Queue__jki_lib_state_machine.vi"("State(s) in (\"\")"=w272) -> ("States Out"=w271:string)  [unwired: 14 in]
      }
      frame "Macro: Initialize" {
        w276 = "Data: Initialize\nInit: Time\nInitialize Core Data\nUI: Initialize\nUI: Front Panel State >> Open"  # Data: Initialize Init: Time Initialize Core Data UI: Initialize UI: Front Panel State >> Open
        # "Initialization Macro\n(This is called once, when the VI starts)"
        n101 = call <vilib>:"Add State(s) to Queue__jki_lib_state_machine.vi"("State(s) in Front (\"\")"=w276, "State(s) in (\"\")"=w280) -> ("States Out"=w279:string)  [unwired: 13 in]
      }
      frame "Macro: Exit" {
        # "Exit Macro\n(This is called once, when the VI exits)"
        n102 = Unbundle By Name(w290) -> ("Core.Close Panel on Exit?"=w289:bool)
        n103 = Select(t="UI: Front Panel State >> Close", s=w289, f="") -> (s? t:f=w286:string)
        n104 = call <vilib>:"Add State(s) to Queue__jki_lib_state_machine.vi"("State(s) in (\"\")"=w286, "State(s) at Back (\"\")"="Data: Cleanup\nInit: Power Analyzer kWatts\nExit") -> ("States Out"=w284:string)  [unwired: 13 in]
        n105 = call <vilib>:"Add State(s) to Queue__jki_lib_state_machine.vi"("State(s) in Front (\"\")"=w284, "State(s) in (\"\")"=w293) -> ("States Out"=w292:string)  [unwired: 13 in]
      }
      frame "----Initialize Equipment----" {
        # "Template Separator\n(You can make a copy of, or modify, this frame)"
        n106 = call <vilib>:"Add State(s) to Queue__jki_lib_state_machine.vi"("State(s) in (\"\")"=w300) -> ("States Out"=w299:string)  [unwired: 14 in]
      }
      frame "Init: Power Analyzer Watts" {
        # "Template Separator\n(You can make a copy of, or modify, this frame)"
        n107 = Unbundle By Name(w310) -> ("Equipment.Com Power Meter"=w309:refnum<visa-resource-name>)
        n108 = local read "Testing"() -> (w304:bool)
        n109 = case shown="False" w304 {
          tunnel: w309 -> [w320 _]
          tunnel: [w316 w321] -> w303
          tunnel: w308 -> [w315 w321]
          frame False {
            w318 = u16 3 items=["AUTO", "500 mA", "1 A", "2 A", "5 A", "10 A", "20 A", "40 A", "S-AUTO", "50 mV", "100 mV", "200 mV", "500 mV", "1 V", "2 V", "5 V", "10 V", "250 mA", "500 mA", "1 A", "2.5 A", "5 A", "10 A", "20 A", "25 mV", "50 mV", "100 mV", "250 mV", "500 mV", "1 V", "2.5 V", "5 V"] ("I Range (7: 40A)")
            w319 = u16 6 items=["AUTO", "15", "30", "60", "100", "150", "300", "600", "1000", "7.5", "15", "30", "50", "75", "150", "300", "500"] ("V Range (8: 1000V)")
            n110 = call "WT500 Read Power.vi"("VISA resource name"=w320, "WT500 CMDS"=WT500_Sequences."Initialize", "V Range (8: 1000V)"=w319, "I Range (7: 40A)"=w318, "error in (no error)"=w315) -> ("error out"=w316:errorcluster)  [unwired: 5 in, 5 out]
          }
          frame True {
          }
        }
        n111 = call "Delay mS.vi"("Error In"=w303, "milliseconds to wait"=u32 3000) -> ("Error Out"=w302:errorcluster)  [unwired: 13 in]
        n112 = case shown="No Error" w302 {
          tunnel: ["" ("State(s) in Front (\"\")") "Macro: Exit" ("State(s) in Front (\"\")")] -> w306
          tunnel: w307 -> [_ w324]
          frame No Error {
          }
          frame Error {
            n113 = Concatenate Strings("Error:", w324) -> (w326:string)
            n114 = One Button Dialog(message=w326) -> ()  [unwired: 1 in, 1 out]
          }
        }
        n115 = call <vilib>:"Add State(s) to Queue__jki_lib_state_machine.vi"("State(s) in Front (\"\")"=w306, "State(s) in (\"\")"=w314) -> ("States Out"=w313:string)  [unwired: 13 in]
      }
      frame "Init: Power Analyzer kWatts" {
        # "Template Separator\n(You can make a copy of, or modify, this frame)"
        n116 = Unbundle By Name(w336) -> ("Equipment.Com Power Meter"=w335:refnum<visa-resource-name>)
        n117 = local read "Testing"() -> (w330:bool)
        n118 = case shown="False" w330 {
          tunnel: w335 -> [w346 _]
          tunnel: [w342 w347] -> w329
          tunnel: w334 -> [w341 w347]
          frame False {
            w344 = u16 7 items=["AUTO", "500 mA", "1 A", "2 A", "5 A", "10 A", "20 A", "40 A", "S-AUTO", "50 mV", "100 mV", "200 mV", "500 mV", "1 V", "2 V", "5 V", "10 V", "250 mA", "500 mA", "1 A", "2.5 A", "5 A", "10 A", "20 A", "25 mV", "50 mV", "100 mV", "250 mV", "500 mV", "1 V", "2.5 V", "5 V"] ("I Range (7: 40A)")
            w345 = u16 6 items=["AUTO", "15", "30", "60", "100", "150", "300", "600", "1000", "7.5", "15", "30", "50", "75", "150", "300", "500"] ("V Range (8: 1000V)")
            n119 = call "WT500 Read Power.vi"("VISA resource name"=w346, "WT500 CMDS"=WT500_Sequences."Initialize", "V Range (8: 1000V)"=w345, "I Range (7: 40A)"=w344, "error in (no error)"=w341) -> ("error out"=w342:errorcluster)  [unwired: 5 in, 5 out]
          }
          frame True {
          }
        }
        n120 = call "Delay mS.vi"("Error In"=w329, "milliseconds to wait"=u32 3000) -> ("Error Out"=w328:errorcluster)  [unwired: 13 in]
        n121 = case shown="No Error" w328 {
          tunnel: ["" ("State(s) in Front (\"\")") "Macro: Exit" ("State(s) in Front (\"\")")] -> w332
          tunnel: w333 -> [_ w350]
          frame No Error {
          }
          frame Error {
            n122 = Concatenate Strings("Error:", w350) -> (w352:string)
            n123 = One Button Dialog(message=w352) -> ()  [unwired: 1 in, 1 out]
          }
        }
        n124 = call <vilib>:"Add State(s) to Queue__jki_lib_state_machine.vi"("State(s) in Front (\"\")"=w332, "State(s) in (\"\")"=w340) -> ("States Out"=w339:string)  [unwired: 13 in]
      }
      frame "----------Test ----------" {
        # "Template Separator\n(You can make a copy of, or modify, this frame)"
        n125 = call <vilib>:"Add State(s) to Queue__jki_lib_state_machine.vi"("State(s) in (\"\")"=w359) -> ("States Out"=w358:string)  [unwired: 14 in]
      }
      frame "Get Power Threshold" {
        # "Your code here.\n(You can make a copy of, or modify, this frame)"
        n126 = Unbundle By Name(w373) -> ("Tstart"=w370:dbl, "2015?"=w366:bool, "35 Min Data Array"=w365:dbl[])
        n127 = Build Array (concatenate)(w361, w365) -> (w360:dbl[][])
        "Power Threshold Array" <- w360
        n128 = local read "Timer"() -> (w368:dbl)
        n129 = Greater?(x=w368, y=30.0) -> (0:w369:bool)
        n130 = case shown="False" w369 {
          tunnel: w373 -> [w384 w394]
          tunnel: [w383 w393] -> w372
          tunnel: [w382 "" ("State(s) in Front (\"\")")] -> w371
          tunnel: w370 -> [w379 _]
          tunnel: w366 -> [w378 _]
          tunnel: w360 -> [_ w402]
          frame False {
            n131 = call "E-Time.vi"() -> ("Elapsed Time (sec)"=w385:dbl)  [unwired: 9 in, 2 out]
            n132 = call "RLT Timeout Calc.vi"("Complete time"=w385, "Gather Data Period"=1000, "Start Time"=w379) -> ("coerced(x)"=w381:i32)  [unwired: 8 in]
            n133 = event shown="[0] Timeout" {
              selector: _ -> [_]
              dyn-events: _ -> [_]
              timeout: w381 -> [_]
              tunnel: [w388] -> w377
              tunnel: [w387] -> w382
              tunnel: w378 -> [w386]
              event Timeout {
                n134 = event-data() -> ()  [unwired: 1 in, 2 out]
                n135 = case shown="True" w386 {
                  tunnel: ["Post Time\nGet Power\nGet Power Threshold" ("State(s) in Front (\"\")") "Post Time\nGet Power\nAgilent: Get Data\nWait for 5 Mins" ("State(s) in Front (\"\")")] -> w387
                  frame True {
                  }
                  frame False {
                  }
                }
                n136 = call "E-Time.vi"() -> ("Elapsed Time (sec)"=w388:dbl)  [unwired: 9 in, 2 out]
              }
            }
            n137 = Bundle By Name(cluster=w384, "Tstart"=w377) -> (w383:T8)
          }
          frame True {
            # "Set the Power Threshold at 150% of the average"
            n138 = Delete From Array(array=w402, index (col)=1 ("disabled index (col)")) -> (deleted portion=w397:dbl[])  [unwired: 2 in, 1 out]
            n139 = Delete From Array(array=w397, index=0) -> (array with subset deleted=w395:dbl[])  [unwired: 1 in, 1 out]
            n140 = call <vilib>:"Std Deviation and Variance.vi"("X"=w395) -> ("mean"=w400:dbl)  [unwired: 1 in, 2 out]
            n141 = call "E-Time.vi"("Reset"=TRUE) -> ("Elapsed Time (sec)"=w392:dbl)  [unwired: 8 in, 2 out]
            n142 = Multiply(x=w400, y=1.5) -> (x*y=→"Power Threshold":dbl)
            n143 = Bundle By Name(cluster=w394, "Tstart"=w392, "T0"=w392) -> (w393:T8)
          }
        }
        n144 = local write "String"("Calculating the Power Threshold...") -> ()
        n145 = call <vilib>:"Add State(s) to Queue__jki_lib_state_machine.vi"("State(s) in Front (\"\")"=w371, "State(s) in (\"\")"=w376) -> ("States Out"=w375:string)  [unwired: 13 in]
      }
      frame "Wait for Power On" {
        # "Your code here.\n(You can make a copy of, or modify, this frame)"
        n146 = local read "Power (Watts)"() -> (w411:dbl)
        n147 = local read "Power Threshold"() -> (w405:dbl)
        n148 = Unbundle By Name(w415) -> ("2015?"=w409:bool, "Tstart"=w412:dbl)
        n149 = Greater?(x=w405, y=w411) -> (0:w410:bool)
        n150 = case shown="True" w410 {
          tunnel: w415 -> [w421 w430]
          tunnel: [w421 w429] -> w414
          tunnel: ["" ("State(s) in Front (\"\")") w427] -> w413
          tunnel: w412 -> [_ w424]
          tunnel: w409 -> [_ w422]
          frame False {
            n151 = local write "Timer"(0.0 ("Timer")) -> ()
          }
          frame True {
            n152 = call "E-Time.vi"() -> ("Elapsed Time (sec)"=w431:dbl)  [unwired: 9 in, 2 out]
            n153 = call "RLT Timeout Calc.vi"("Complete time"=w431, "Gather Data Period"=1000, "Start Time"=w424) -> ("coerced(x)"=w426:i32)  [unwired: 8 in]
            n154 = event shown="[0] Timeout" {
              selector: _ -> [_]
              dyn-events: _ -> [_]
              timeout: w426 -> [_]
              tunnel: [w433] -> w428
              tunnel: [w434] -> w427
              tunnel: [w433] -> w423
              tunnel: w422 -> [w432]
              event Timeout {
                n155 = event-data() -> ()  [unwired: 1 in, 2 out]
                n156 = case shown="True" w432 {
                  tunnel: ["Get Power\nWait for Power On" ("State(s) in Front (\"\")") "Get Power\nAgilent: Get Data\nWait for Power On" ("State(s) in Front (\"\")")] -> w434
                  frame True {
                  }
                  frame False {
                  }
                }
                n157 = call "E-Time.vi"() -> ("Elapsed Time (sec)"=w433:dbl)  [unwired: 9 in, 2 out]
              }
            }
            n158 = Bundle By Name(cluster=w430, "Tstart"=w428, "T0"=w423) -> (w429:T8)
          }
        }
        n159 = call <vilib>:"Add State(s) to Queue__jki_lib_state_machine.vi"("State(s) in Front (\"\")"=w413, "State(s) in (\"\")"=w418) -> ("States Out"=w417:string)  [unwired: 13 in]
        "String" <- "Waiting for Power ON"
      }
      frame "High State" {
        # "Your code here.\n(You can make a copy of, or modify, this frame)"
        n160 = Unbundle By Name(w449) -> ("Tstart"=w446:dbl, "2015?"=w442:bool)
        n161 = local read "Timer"() -> (w444:dbl)
        n162 = Greater?(x=w444, y="High State Timer") -> (0:w445:bool)
        n163 = case shown="True" w445 {
          tunnel: w449 -> [w461 w470]
          tunnel: [w460 w470] -> w448
          tunnel: [w458 "" ("State(s) in Front (\"\")")] -> w447
          tunnel: w446 -> [w455 _]
          tunnel: w442 -> [w454 _]
          tunnel: string[] ["Time", "Power", "Ambient Temp (F)", "RH", "RDB (F)"] ("Array") -> [w453 _]
          frame False {
            n164 = call "E-Time.vi"() -> ("Elapsed Time (sec)"=w462:dbl)  [unwired: 9 in, 2 out]
            n165 = call "RLT Timeout Calc.vi"("Complete time"=w462, "Gather Data Period"=1000, "Start Time"=w455) -> ("coerced(x)"=w457:i32)  [unwired: 8 in]
            n166 = event shown="[0] Timeout" {
              selector: _ -> [_]
              dyn-events: _ -> [_]
              timeout: w457 -> [_]
              tunnel: [w465] -> w459
              tunnel: [w464] -> w458
              tunnel: w454 -> [w463]
              event Timeout {
                n167 = event-data() -> ()  [unwired: 1 in, 2 out]
                n168 = case shown="True" w463 {
                  tunnel: ["Post Time\nGet Power\nHigh State" ("State(s) in Front (\"\")") "Post Time\nGet Power\nAgilent: Get Data\nWait for 5 Mins" ("State(s) in Front (\"\")")] -> w464
                  frame True {
                  }
                  frame False {
                  }
                }
                n169 = call "E-Time.vi"() -> ("Elapsed Time (sec)"=w465:dbl)  [unwired: 9 in, 2 out]
              }
            }
            n170 = Bundle By Name(cluster=w461, "Tstart"=w459, "Labels"=w453) -> (w460:T8)
          }
          frame True {
            # "Set the high power state"
            n171 = local read "Power (Watts)"() -> (→"High Power":dbl)
          }
        }
        n172 = local write "String"("Recording High Power State...") -> ()
        n173 = call <vilib>:"Add State(s) to Queue__jki_lib_state_machine.vi"("State(s) in Front (\"\")"=w447, "State(s) in (\"\")"=w452) -> ("States Out"=w451:string)  [unwired: 13 in]
      }
      frame "Check for Low Power" {
        # "Your code here.\n(You can make a copy of, or modify, this frame)"
        n174 = Unbundle By Name(w486) -> ("Tstart"=w483:dbl, "2015?"=w479:bool, "Low Power State?"=w473:bool)
        n175 = local read "High State Timer"() -> (w475:dbl)
        n176 = local read "Timer"() -> (w481:dbl)
        n177 = Add(x="Low State Timer (5 min)", y=w475) -> (x+y=w474:dbl)
        "Time Sum 1" <- w474
        n178 = Greater?(x=w481, y=w474) -> (0:w482:bool)
        n179 = case shown="False" w473 {
          tunnel: w486 -> [w496 w515]
          tunnel: [w495 w515] -> w485
          tunnel: [w494 "Wait for 35 Mins\nWait for 10 Mins\nData Process"] -> w484
          tunnel: w483 -> [w493 _]
          tunnel: w482 -> [w492 _]
          tunnel: w479 -> [w491 _]
          tunnel: string[] ["Time", "Power", "Ambient Temp (F)", "RH", "RDB (F)"] ("Array") -> [w490 _]
          frame False {
            n180 = case shown="False" w492 {
              tunnel: w496 -> [w505 w514]
              tunnel: [w504 w514] -> w495
              tunnel: [w502 "Wait 5 Min\nStabilize 5 Min\nOff Mode Collect 5 Min\nData Process" ("State(s) in Front (\"\")")] -> w494
              tunnel: w493 -> [w499 _]
              tunnel: w491 -> [w498 _]
              tunnel: w490 -> [w497 _]
              frame False {
                n181 = call "E-Time.vi"() -> ("Elapsed Time (sec)"=w506:dbl)  [unwired: 9 in, 2 out]
                n182 = call "RLT Timeout Calc.vi"("Complete time"=w506, "Gather Data Period"=1000, "Start Time"=w499) -> ("coerced(x)"=w501:i32)  [unwired: 8 in]
                n183 = event shown="[0] Timeout" {
                  selector: _ -> [_]
                  dyn-events: _ -> [_]
                  timeout: w501 -> [_]
                  tunnel: [w509] -> w503
                  tunnel: [w508] -> w502
                  tunnel: w498 -> [w507]
                  event Timeout {
                    n184 = event-data() -> ()  [unwired: 1 in, 2 out]
                    n185 = case shown="True" w507 {
                      tunnel: ["Post Time\nGet Power\nCheck for Low Power" ("State(s) in Front (\"\")") "" ("State(s) in Front (\"\")")] -> w508
                      frame True {
                      }
                      frame False {
                      }
                    }
                    n186 = call "E-Time.vi"() -> ("Elapsed Time (sec)"=w509:dbl)  [unwired: 9 in, 2 out]
                  }
                }
                n187 = Bundle By Name(cluster=w505, "Tstart"=w503, "Labels"=w497) -> (w504:T8)
              }
              frame True {
                n188 = local write "Low Power Switch"(FALSE ("Low Power Switch")) -> ()
              }
            }
          }
          frame True {
          }
        }
        n189 = local write "String"("Checking for a Low Power State...") -> ()
        n190 = call <vilib>:"Add State(s) to Queue__jki_lib_state_machine.vi"("State(s) in Front (\"\")"=w484, "State(s) in (\"\")"=w489) -> ("States Out"=w488:string)  [unwired: 13 in]
      }
      frame "Wait 5 Min" {
        # "Your code here.\n(You can make a copy of, or modify, this frame)"
        n191 = Unbundle By Name(w533) -> ("Tstart"=w530:dbl, "2015?"=w526:bool, "35 Min Data Array"=w524:dbl[])
        n192 = local read "Time Sum 1"() -> (w520:dbl)
        n193 = local read "Timer"() -> (w528:dbl)
        n194 = Add(x=w520, y="5 Min Timer") -> (x+y=w523:dbl)
        "Time Sum 3" <- w523
        n195 = Greater?(x=w528, y=w523) -> (0:w529:bool)
        n196 = Build Array (concatenate)(w518, w524) -> (w521:dbl[][])
        n197 = case shown="False" w529 {
          tunnel: w533 -> [w545 w556]
          tunnel: [w544 w556] -> w532
          tunnel: [w542 w552] -> w531
          tunnel: w530 -> [w539 _]
          tunnel: w526 -> [w538 _]
          tunnel: string[] ["Time", "Power", "Ambient Temp (F)", "RH", "RDB (F)"] ("Array") -> [w537 _]
          frame False {
            n198 = call "E-Time.vi"() -> ("Elapsed Time (sec)"=w546:dbl)  [unwired: 9 in, 2 out]
            n199 = call "RLT Timeout Calc.vi"("Complete time"=w546, "Gather Data Period"=1000, "Start Time"=w539) -> ("coerced(x)"=w541:i32)  [unwired: 8 in]
            n200 = event shown="[0] Timeout" {
              selector: _ -> [_]
              dyn-events: _ -> [_]
              timeout: w541 -> [_]
              tunnel: [w549] -> w543
              tunnel: [w548] -> w542
              tunnel: w538 -> [w547]
              event Timeout {
                n201 = event-data() -> ()  [unwired: 1 in, 2 out]
                n202 = case shown="True" w547 {
                  tunnel: ["Post Time\nGet Power\nWait 5 Min" ("State(s) in Front (\"\")") "" ("State(s) in Front (\"\")")] -> w548
                  frame True {
                  }
                  frame False {
                  }
                }
                n203 = call "E-Time.vi"() -> ("Elapsed Time (sec)"=w549:dbl)  [unwired: 9 in, 2 out]
              }
            }
            n204 = Bundle By Name(cluster=w545, "Tstart"=w543, "Labels"=w537) -> (w544:T8)
          }
          frame True {
            n205 = One Button Dialog(message="Turn Dryer Off", button name ("OK")="OK") -> (true=w553:bool)
            n206 = case shown="True" w553 {
              tunnel: ["Macro: Exit" ("State(s) in Front (\"\")") "" ("State(s) in Front (\"\")")] -> w552
              frame False {
              }
              frame True {
              }
            }
          }
        }
        n207 = local write "DOE Data"(w521) -> ()
        n208 = call <vilib>:"Add State(s) to Queue__jki_lib_state_machine.vi"("State(s) in Front (\"\")"=w531, "State(s) in (\"\")"=w536) -> ("States Out"=w535:string)  [unwired: 13 in]
        n209 = local write "String"("Collecting Standby Data For 5 Min...") -> ()
      }
      frame "Stabilize 5 Min" {
        # "Your code here.\n(You can make a copy of, or modify, this frame)"
        n210 = local read "Time Sum 3"() -> (w562:dbl)
        n211 = local read "5 Min Timer"() -> (w560:dbl)
        n212 = Unbundle By Name(w573) -> ("Tstart"=w570:dbl, "2015?"=w566:bool)
        n213 = local read "Timer"() -> (w568:dbl)
        n214 = Add(x=w562, y=w560) -> (x+y=w564:dbl)
        "Time Sum 4" <- w564
        n215 = Greater?(x=w568, y=w564) -> (0:w569:bool)
        n216 = case shown="False" w569 {
          tunnel: w573 -> [w585 w593]
          tunnel: [w584 w593] -> w572
          tunnel: [w582 "" ("State(s) in Front (\"\")")] -> w571
          tunnel: w570 -> [w579 _]
          tunnel: w566 -> [w578 _]
          tunnel: string[] ["Time", "Power", "Ambient Temp (F)", "RH", "RDB (F)"] ("Array") -> [w577 _]
          frame False {
            n217 = call "E-Time.vi"() -> ("Elapsed Time (sec)"=w586:dbl)  [unwired: 9 in, 2 out]
            n218 = call "RLT Timeout Calc.vi"("Complete time"=w586, "Gather Data Period"=1000, "Start Time"=w579) -> ("coerced(x)"=w581:i32)  [unwired: 8 in]
            n219 = event shown="[0] Timeout" {
              selector: _ -> [_]
              dyn-events: _ -> [_]
              timeout: w581 -> [_]
              tunnel: [w589] -> w583
              tunnel: [w588] -> w582
              tunnel: w578 -> [w587]
              event Timeout {
                n220 = event-data() -> ()  [unwired: 1 in, 2 out]
                n221 = case shown="True" w587 {
                  tunnel: ["Post Time\nGet Power\nStabilize 5 Min" ("State(s) in Front (\"\")") "" ("State(s) in Front (\"\")")] -> w588
                  frame True {
                  }
                  frame False {
                  }
                }
                n222 = call "E-Time.vi"() -> ("Elapsed Time (sec)"=w589:dbl)  [unwired: 9 in, 2 out]
              }
            }
            n223 = Bundle By Name(cluster=w585, "Tstart"=w583, "Labels"=w577) -> (w584:T8)
          }
          frame True {
          }
        }
        n224 = call <vilib>:"Add State(s) to Queue__jki_lib_state_machine.vi"("State(s) in Front (\"\")"=w571, "State(s) in (\"\")"=w576) -> ("States Out"=w575:string)  [unwired: 13 in]
        n225 = local write "String"("Stabilizing for 5 Min...") -> ()
      }
      frame "Off Mode Collect 5 Min" {
        # "Your code here.\n(You can make a copy of, or modify, this frame)"
        n226 = Unbundle By Name(w610) -> ("Tstart"=w607:dbl, "2015?"=w603:bool, "35 Min Data Array"=w600:dbl[])
        n227 = Build Array (concatenate)(w601, w600) -> (w596:dbl[][])
        n228 = local read "5 Min Timer"() -> (w595:dbl)
        n229 = local read "Time Sum 4"() -> (w598:dbl)
        n230 = local write "35 Min Data"(w596) -> ()
        n231 = local read "Timer"() -> (w605:dbl)
        n232 = Add(x=w595, y=w598) -> (x+y=w597:dbl)
        n233 = Greater?(x=w605, y=w597) -> (0:w606:bool)
        n234 = case shown="False" w606 {
          tunnel: w610 -> [w622 w630]
          tunnel: [w621 w630] -> w609
          tunnel: [w619 "" ("State(s) in Front (\"\")")] -> w608
          tunnel: w607 -> [w616 _]
          tunnel: w603 -> [w615 _]
          tunnel: string[] ["Time", "Power", "Ambient Temp (F)", "RH", "RDB (F)"] ("Array") -> [w614 _]
          frame False {
            n235 = call "E-Time.vi"() -> ("Elapsed Time (sec)"=w623:dbl)  [unwired: 9 in, 2 out]
            n236 = call "RLT Timeout Calc.vi"("Complete time"=w623, "Gather Data Period"=1000, "Start Time"=w616) -> ("coerced(x)"=w618:i32)  [unwired: 8 in]
            n237 = event shown="[0] Timeout" {
              selector: _ -> [_]
              dyn-events: _ -> [_]
              timeout: w618 -> [_]
              tunnel: [w626] -> w620
              tunnel: [w625] -> w619
              tunnel: w615 -> [w624]
              event Timeout {
                n238 = event-data() -> ()  [unwired: 1 in, 2 out]
                n239 = case shown="True" w624 {
                  tunnel: ["Post Time\nGet Power\nOff Mode Collect 5 Min" ("State(s) in Front (\"\")") "Post Time\nGet Power\nAgilent: Get Data\nWait for 5 Mins" ("State(s) in Front (\"\")")] -> w625
                  frame True {
                  }
                  frame False {
                  }
                }
                n240 = call "E-Time.vi"() -> ("Elapsed Time (sec)"=w626:dbl)  [unwired: 9 in, 2 out]
              }
            }
            n241 = Bundle By Name(cluster=w622, "Tstart"=w620, "Labels"=w614) -> (w621:T8)
          }
          frame True {
          }
        }
        n242 = local write "String"("Collecting Off Mode Watts...") -> ()
        n243 = call <vilib>:"Add State(s) to Queue__jki_lib_state_machine.vi"("State(s) in Front (\"\")"=w608, "State(s) in (\"\")"=w613) -> ("States Out"=w612:string)  [unwired: 13 in]
      }
      frame "Wait for 35 Mins" {
        # "Your code here.\n(You can make a copy of, or modify, this frame)"
        n244 = Unbundle By Name(w647) -> ("Tstart"=w644:dbl, "2015?"=w640:bool, "35 Min Data Array"=w637:dbl[])
        n245 = Build Array (concatenate)(w638, w637) -> (w636:dbl[][])
        "35 Min Data" <- w636
        n246 = local read "Time Sum 1"() -> (w633:dbl)
        n247 = Add(x="35 Min", y=w633) -> (x+y=w632:dbl)
        "Time Sum 2" <- w632
        n248 = local read "Timer"() -> (w642:dbl)
        n249 = Greater?(x=w642, y=w632) -> (0:w643:bool)
        n250 = case shown="False" w643 {
          tunnel: w647 -> [w659 w667]
          tunnel: [w658 w667] -> w646
          tunnel: [w656 "" ("State(s) in Front (\"\")")] -> w645
          tunnel: w644 -> [w653 _]
          tunnel: w640 -> [w652 _]
          tunnel: string[] ["Time", "Power", "Ambient Temp (F)", "RH", "RDB (F)"] ("Array") -> [w651 _]
          frame False {
            n251 = call "E-Time.vi"() -> ("Elapsed Time (sec)"=w660:dbl)  [unwired: 9 in, 2 out]
            n252 = call "RLT Timeout Calc.vi"("Complete time"=w660, "Gather Data Period"=1000, "Start Time"=w653) -> ("coerced(x)"=w655:i32)  [unwired: 8 in]
            n253 = event shown="[0] Timeout" {
              selector: _ -> [_]
              dyn-events: _ -> [_]
              timeout: w655 -> [_]
              tunnel: [w663] -> w657
              tunnel: [w662] -> w656
              tunnel: w652 -> [w661]
              event Timeout {
                n254 = event-data() -> ()  [unwired: 1 in, 2 out]
                n255 = case shown="True" w661 {
                  tunnel: ["Post Time\nGet Power\nWait for 35 Mins" ("State(s) in Front (\"\")") "Post Time\nGet Power\nAgilent: Get Data\nWait for 5 Mins" ("State(s) in Front (\"\")")] -> w662
                  frame True {
                  }
                  frame False {
                  }
                }
                n256 = call "E-Time.vi"() -> ("Elapsed Time (sec)"=w663:dbl)  [unwired: 9 in, 2 out]
              }
            }
            n257 = Bundle By Name(cluster=w659, "Tstart"=w657, "Labels"=w651) -> (w658:T8)
          }
          frame True {
          }
        }
        n258 = local write "String"("Off Mode Stabilization...") -> ()
        n259 = call <vilib>:"Add State(s) to Queue__jki_lib_state_machine.vi"("State(s) in Front (\"\")"=w645, "State(s) in (\"\")"=w650) -> ("States Out"=w649:string)  [unwired: 13 in]
      }
      frame "Wait for 10 Mins" {
        # "Your code here.\n(You can make a copy of, or modify, this frame)"
        n260 = Unbundle By Name(w684) -> ("Tstart"=w681:dbl, "2015?"=w677:bool, "35 Min Data Array"=w675:dbl[])
        n261 = Build Array (concatenate)(w674, w675) -> (w673:dbl[][])
        "DOE Data" <- w673
        n262 = local read "Time Sum 2"() -> (w670:dbl)
        n263 = local read "Timer"() -> (w679:dbl)
        n264 = Add(x="10 Min Power", y=w670) -> (x+y=w671:dbl)
        n265 = Greater?(x=w679, y=w671) -> (0:w680:bool)
        n266 = case shown="False" w680 {
          tunnel: w684 -> [w696 w704]
          tunnel: [w695 w704] -> w683
          tunnel: [w693 "" ("State(s) in Front (\"\")")] -> w682
          tunnel: w681 -> [w690 _]
          tunnel: w677 -> [w689 _]
          tunnel: string[] ["Time", "Power", "Ambient Temp (F)", "RH", "RDB (F)"] ("Array") -> [w688 _]
          frame False {
            n267 = call "E-Time.vi"() -> ("Elapsed Time (sec)"=w697:dbl)  [unwired: 9 in, 2 out]
            n268 = call "RLT Timeout Calc.vi"("Complete time"=w697, "Gather Data Period"=1000, "Start Time"=w690) -> ("coerced(x)"=w692:i32)  [unwired: 8 in]
            n269 = event shown="[0] Timeout" {
              selector: _ -> [_]
              dyn-events: _ -> [_]
              timeout: w692 -> [_]
              tunnel: [w700] -> w694
              tunnel: [w699] -> w693
              tunnel: w689 -> [w698]
              event Timeout {
                n270 = event-data() -> ()  [unwired: 1 in, 2 out]
                n271 = case shown="True" w698 {
                  tunnel: ["Post Time\nGet Power\nWait for 10 Mins" ("State(s) in Front (\"\")") "Post Time\nGet Power\nAgilent: Get Data\nWait for 5 Mins" ("State(s) in Front (\"\")")] -> w699
                  frame True {
                  }
                  frame False {
                  }
                }
                n272 = call "E-Time.vi"() -> ("Elapsed Time (sec)"=w700:dbl)  [unwired: 9 in, 2 out]
              }
            }
            n273 = Bundle By Name(cluster=w696, "Tstart"=w694, "Labels"=w688) -> (w695:T8)
          }
          frame True {
          }
        }
        n274 = local write "String"("Collecting Data For 10 Min...") -> ()
        n275 = call <vilib>:"Add State(s) to Queue__jki_lib_state_machine.vi"("State(s) in Front (\"\")"=w682, "State(s) in (\"\")"=w687) -> ("States Out"=w686:string)  [unwired: 13 in]
      }
      frame "Data Process" {
        # "Your code here.\n(You can make a copy of, or modify, this frame)"
        n276 = Unbundle By Name(w706) -> ("Output Data"=w725:T9)
        n277 = local read "Low Power Switch"() -> (w712:bool)
        n278 = case shown="True" w712 {
          tunnel: [w743 w761] -> w730
          tunnel: [w745 w766] -> w729
          tunnel: [w740 w761] -> w728
          tunnel: [w742 w761] -> w727
          tunnel: [w741 w761] -> w726
          tunnel: [w748 w765] -> w710
          tunnel: [w744 w764] -> w724
          tunnel: [w746 w763] -> w723
          tunnel: [w747 w762] -> w722
          frame False {
            # "Due to the order of the state machine, \nI had to switch the order of the  standby\nand off mode values."
            n279 = local read "DOE Data"() -> (w755:dbl[][])
            n280 = local read "35 Min Data"() -> (w756:dbl[][])
            n281 = Delete From Array(array=w755, index (col)=1 ("disabled index (col)")) -> (deleted portion=w752:dbl[])  [unwired: 2 in, 1 out]
            n282 = Delete From Array(array=w756, index (col)=1 ("disabled index (col)")) -> (deleted portion=w760:dbl[])  [unwired: 2 in, 1 out]
            n283 = call <vilib>:"Histogram.vi"("X"=w752) -> ("Histogram Graph"=w751:T1)  [unwired: 7 in, 3 out]
            n284 = call <vilib>:"Std Deviation and Variance.vi"("X"=w752) -> ("mean"=w743:dbl, "standard deviation"=w740:dbl)  [unwired: 1 in, 1 out]
            n285 = Array Max & Min(array=w752) -> (max value=w742:dbl)  [unwired: 3 out]
            n286 = call <vilib>:"Histogram.vi"("X"=w760) -> ("Histogram Graph"=→"Standby Mode Watts":T1)  [unwired: 7 in, 3 out]
            n287 = call <vilib>:"Std Deviation and Variance.vi"("X"=w760) -> ("mean"=w745:dbl, "standard deviation"=w744:dbl)  [unwired: 1 in, 1 out]
            n288 = Array Max & Min(array=w760) -> (max value=w746:dbl)  [unwired: 3 out]
            n289 = local write "Off Mode Watts"(w751) -> ()
            n290 = Multiply(x=w742, y=0.05) -> (x*y=w741:dbl)
            n291 = Multiply(x=w746, y=0.05) -> (x*y=w747:dbl)
            n292 = Less?(x=w740, y=w741) -> (x < y?=w750:bool)
            n293 = Less?(x=w744, y=w747) -> (x < y?=w749:bool)
            n294 = And(x=w750, y=w749) -> (x .and. y?=w748:bool)
          }
          frame True {
            w761 = 0.0
            n295 = local read "DOE Data"() -> (w771:dbl[][])
            n296 = Delete From Array(array=w771, index (col)=1 ("disabled index (col)")) -> (deleted portion=w767:dbl[])  [unwired: 2 in, 1 out]
            n297 = call <vilib>:"Std Deviation and Variance.vi"("X"=w767) -> ("mean"=w766:dbl, "standard deviation"=w764:dbl)  [unwired: 1 in, 1 out]
            n298 = Array Max & Min(array=w767) -> (max value=w763:dbl)  [unwired: 3 out]
            n299 = call <vilib>:"Histogram.vi"("X"=w767) -> ("Histogram Graph"=→"Off Mode Watts":T1)  [unwired: 7 in, 3 out]
            n300 = Multiply(x=w763, y=0.05) -> (x*y=w762:dbl)
            n301 = Less?(x=w764, y=w762) -> (x < y?=w765:bool)
          }
        }
        "Stable?" <- w710
        n302 = Bundle By Name(cluster=w725, "Standard Deviation"=w728, "Off Mode Watts"=w729, "Standby Watts"=w730, "Max Value"=w727, "5% of Max"=w726, "Standard Deviation."=w724, "Max Value."=w723, "5% of Max."=w722) -> (w721:T9)
        n303 = Unbundle By Name(w721) -> ("Off Mode Watts"=→"Off Mode Watts":dbl, "Standard Deviation."=→"Standard Deviation.":dbl, "Max Value."=→"Max Value.":dbl, "5% of Max."=→"5% of Max.":dbl, "Standby Watts"=→"Standby Watts":dbl, "Standard Deviation"=→"Standard Deviation":dbl, "Max Value"=→"Max Value":dbl, "5% of Max"=→"5% of Max":dbl)
        n304 = local write "Main Tab"(enum32{"Collecting", "Analyzed"}."Analyzed" ("Main Tab")) -> ()
        n305 = Equal?(x=w710, y=FALSE) -> (x = y?=w708:bool)
        n306 = local write "Processed Data"(TRUE ("Processed Data")) -> ()
        n307 = case shown="False" w708 {
          frame False {
            n308 = property on="Complete Test" class="Bool (strict)"("Visible"=TRUE) -> ()  [unwired: 2 in, 2 out]
          }
          frame True {
            w739 = TRUE ("Visible")
            n309 = property on="Complete Test" class="Bool (strict)"("Visible"=w739) -> ()  [unwired: 2 in, 2 out]
            n310 = property on="Restart" class="Bool (strict)"("Visible"=w739) -> ()  [unwired: 2 in, 2 out]
          }
        }
        n311 = local write "String"("Processing Data...") -> ()
        n312 = call <vilib>:"Add State(s) to Queue__jki_lib_state_machine.vi"("State(s) in Front (\"\")"="", "State(s) in (\"\")"=w737) -> ("States Out"=w736:string)  [unwired: 13 in]
      }
      frame "Init: Time" {
        # "Your code here.\n(You can make a copy of, or modify, this frame)"
        n313 = call "E-Time.vi"("error in (no error)"=w775) -> ("error out"=w777:errorcluster, "Elapsed Time (sec)"=w778:dbl)  [unwired: 8 in, 1 out]
        n314 = Bundle By Name(cluster=w776, "T0"=w778, "Tstart"=w778) -> (w779:T8)
        n315 = call <vilib>:"Add State(s) to Queue__jki_lib_state_machine.vi"("State(s) in (\"\")"=w781) -> ("States Out"=w780:string)  [unwired: 14 in]
      }
      frame "Get Power" {
        # "If the power drops below\n75% of the High Power.\nConsider that the low\npower state"
        # "Your code here.\n(You can make a copy of, or modify, this frame)"
        n316 = Unbundle By Name(w797) -> ("Equipment.Com Power Meter"=w792:refnum<visa-resource-name>, "35 Min Data Array"=w795:dbl[])
        n317 = case shown="True" "Testing" {
          tunnel: [w804 "Test Power"] -> w787
          tunnel: w792 -> [w802 _]
          tunnel: w791 -> [w801 w806]
          tunnel: [w800 w806] -> w790
          frame False {
            n318 = call "WT500 Read Power.vi"("VISA resource name"=w802, "WT500 CMDS"=WT500_Sequences."GetReadings", "error in (no error)"=w801) -> ("PowerData"=w805:T11, "error out"=w800:errorcluster)  [unwired: 7 in, 4 out]
            n319 = Unbundle By Name(w805) -> ("Power"=w804:dbl)
          }
          frame True {
          }
        }
        "Power (Watts)" <- w787
        "Power Chart" <- w787
        n320 = Build Array (concatenate)(w795, w787) -> (w794:dbl[])
        n321 = local read "High Power"() -> (w783:dbl)
        n322 = call <vilib>:"Add State(s) to Queue__jki_lib_state_machine.vi"("State(s) in (\"\")"=w799) -> ("States Out"=w798:string)  [unwired: 14 in]
        n323 = Multiply(x=w783, y=0.75) -> (x*y=w782:dbl)
        n324 = Less?(x=w787, y=w782) -> (x < y?=w786:bool)
        n325 = Bundle By Name(cluster=w797, "35 Min Data Array"=w794, "Low Power State?"=w786) -> (w796:T8)
      }
      frame "Post Time" {
        # "Your code here.\n(You can make a copy of, or modify, this frame)"
        n326 = Unbundle By Name(w814) -> ("T0"=w816:dbl)
        n327 = call "E-Time.vi"() -> ("Elapsed Time (sec)"=w817:dbl)  [unwired: 9 in, 2 out]
        n328 = Subtract(x=w817, y=w816) -> (x-y=w812:dbl)
        "Timer" <- w812
        n329 = Build Array(w812) -> (w811:dbl[])
        n330 = Bundle By Name(cluster=w814, "35 Min Data Array"=w811) -> (w813:T8)
        n331 = call <vilib>:"Add State(s) to Queue__jki_lib_state_machine.vi"("State(s) in (\"\")"=w819) -> ("States Out"=w818:string)  [unwired: 14 in]
      }
    }
    n332 = case shown="True" "Debug?" {
      tunnel: w36 -> [_ w55]
      tunnel: w34 -> [w52 w54]
      tunnel: [w52 w53] -> w35
      frame False {
      }
      frame True {
        n333 = Build Array (concatenate)(w54, w55) -> (w53:string[])
        "Debug State" <- w53
      }
    }
    n334 = case shown="False" "stop" {
      tunnel: [w47 w51] -> w28
      tunnel: w29 -> [w47 w48]
      frame False {
      }
      frame True {
        n335 = call <vilib>:"Add State(s) to Queue__jki_lib_state_machine.vi"("State(s) in Front (\"\")"="Macro: Exit", "State(s) in (\"\")"=w48) -> ("States Out"=w51:string)  [unwired: 13 in]
        n336 = local write "Skip Standby"(FALSE ("Exit")) -> ()
      }
    }
  }
  "Error Out" <- w5
